vi "Main.vi"() -> ()   [LabVIEW 2017]
doc: "The myRIO Project template acquires acceleration data from the onboard accelerometer and displays the changes of acceleration values in a waveform chart."
uses:
  StateMachineControl.ctl
  <vilib>/Platform/TimedLoop/XDataNode/timing_clust.ctl
  <vilib>/Platform/TimedLoop/XDataNode/nitl_modes.ctl
  <vilib>/Platform/TimedLoop/XDataNode/wakeup.ctl
  <vilib>/robotics/Obstacle Avoidance/Simple Vector Field Histogram/Panic Range.ctl
  <vilib>/myRIO/Instrument Drivers/Onboard IO/DIO/typedefs/DIO Reference.ctl
  <vilib>/myRIO/Common/Instrument Driver Framework/Utilities/typedefs/myRIO Generic Hardware Reference.ctl
  <vilib>/myRIO/Common/Instrument Driver Framework/Utilities/typedefs/Hardware Version Enum.ctl
  <vilib>/myRIO/Common/Instrument Driver Framework/Utilities/typedefs/myRIO v1.0 Reference.ctl
  <vilib>/myRIO/Common/Instrument Driver Framework/Utilities/typedefs/Generic FPGA Reference.ctl
  <vilib>/myRIO/Common/Instrument Driver Framework/myRIO v1.0/DIO/typedefs/DIO Channels List.ctl
  <vilib>/myRIO/Common/Instrument Driver Framework/myRIO v1.0/DIO/typedefs/DIO Channels Enum.ctl
  <vilib>/userdefined/High Color/nirio_resource_hc.ctl
  <vilib>/myRIO/Common/Instrument Driver Framework/myRIO v1.0/Encoder/typedefs/Encoder Signal Mode.ctl
  <vilib>/myRIO/Instrument Drivers/Onboard IO/Encoder/typedefs/Encoder Reference.ctl
  <vilib>/myRIO/Common/Instrument Driver Framework/myRIO v1.0/Encoder/typedefs/Encoder Channels Enum.ctl
  <vilib>/myRIO/Common/Instrument Driver Framework/myRIO v1.0/Encoder/typedefs/Encoder Configuration v1.0.ctl
  <vilib>/myRIO/Instrument Drivers/Onboard IO/PWM/typedefs/PWM Reference.ctl
  <vilib>/myRIO/Common/Instrument Driver Framework/myRIO v1.0/PWM/typedefs/PWM Channels Enum.ctl
  <vilib>/myRIO/Instrument Drivers/Onboard IO/PWM/typedefs/PWM Configuration.ctl
  <vilib>/myRIO/Common/Instrument Driver Framework/Utilities/vis/Is FPGA Ref Available.vi
  <vilib>/myRIO/Common/Instrument Driver Framework/myRIO v1.0/DIO/vis/myRIO v1.1 Open DIO.vi
  <vilib>/myRIO/Instrument Drivers/Onboard IO/DIO/vis/Read.vi
  <vilib>/myRIO/Instrument Drivers/Onboard IO/DIO/vis/Write.vi
  <vilib>/myRIO/Common/Instrument Driver Framework/myRIO v1.0/Encoder/vis/myRIO v1.1 Open Encoder.vi
  <vilib>/myRIO/Instrument Drivers/Onboard IO/Encoder/vis/Read.vi
  <vilib>/myRIO/Common/Instrument Driver Framework/myRIO v1.0/PWM/vis/myRIO v1.1 Open PWM.vi
  <vilib>/myRIO/Instrument Drivers/Onboard IO/PWM/vis/Set Duty Cycle and Frequency.vi
  <vilib>/myRIO/Common/Instrument Driver Framework/Utilities/vis/Validate Channels.vi
  <vilib>/myRIO/Common/Instrument Driver Framework/myRIO v1.0/DIO/vis/myRIO v1.0 Reserve DIO.vi
  <vilib>/myRIO/Common/Instrument Driver Framework/myRIO v1.0/Encoder/vis/myRIO v1.0 Reserve Encoder.vi
  <vilib>/myRIO/Common/Instrument Driver Framework/myRIO v1.0/PWM/vis/myRIO v1.0 Reserve PWM.vi
  <vilib>/myRIO/Common/Instrument Driver Framework/myRIO v1.0/UART/vis/myRIO v1.0 Close UART.vi
  <vilib>/myRIO/Common/Instrument Driver Framework/myRIO v1.0/Resource Manager/vis/myRIO v1.0 Reserve Channel List.vi
  <vilib>/myRIO/Common/Instrument Driver Framework/myRIO v1.0/DIO/vis/myRIO v1.0 Build MUX Configuration DIO.vi
  <vilib>/myRIO/Common/Instrument Driver Framework/myRIO v1.0/Encoder/vis/myRIO v1.0 Build MUX Configuration Encoder.vi
  <vilib>/myRIO/Common/Instrument Driver Framework/myRIO v1.0/PWM/vis/myRIO v1.0 Build MUX Configuration PWM.vi
  <vilib>/myRIO/Common/Instrument Driver Framework/myRIO v1.0/Resource Manager/vis/myRIO v1.0 Reserve Channel.vi
  <vilib>/myRIO/Common/Instrument Driver Framework/myRIO v1.0/Resource Manager/vis/myRIO v1.0 Unreserve Channel.vi
  <vilib>/myRIO/Common/Instrument Driver Framework/myRIO v1.0/Resource Manager/vis/myRIO v1.0 Create Configuration List.vi
  <vilib>/myRIO/Common/Instrument Driver Framework/myRIO v1.0/Resource Manager/vis/myRIO v1.0 Build Mutex Name.vi
  <vilib>/Utility/VariantDataType/GetNumericInfo.vi
  <vilib>/Utility/error.llb/Error Cluster From Error Code.vi
  <vilib>/myRIO/Common/Instrument Driver Framework/myRIO v1.0/myRIO v1.1 Open.vi
  <vilib>/myRIO/Common/Instrument Driver Framework/Utilities/vis/IO Manager.vi
  <vilib>/myRIO/Common/Instrument Driver Framework/Utilities/vis/Configuration Manager.vi
  <vilib>/myRIO/Common/Instrument Driver Framework/myRIO v1.0/Resource Manager/vis/myRIO v1.0 Configure IO.vi
  <vilib>/myRIO/Common/Instrument Driver Framework/myRIO v1.0/myRIO v1.0 Close.vi
  <vilib>/myRIO/Common/Instrument Driver Framework/myRIO v1.0/DIO/vis/myRIO v1.0 Read DIO.vi
  <vilib>/myRIO/Common/Instrument Driver Framework/myRIO v1.0/DIO/vis/myRIO v1.0 Write DIO.vi
  <vilib>/myRIO/Common/Instrument Driver Framework/myRIO v1.0/Encoder/vis/myRIO v1.0 Configure Encoder.vi
  <vilib>/myRIO/Common/Instrument Driver Framework/myRIO v1.0/Encoder/vis/myRIO v1.0 Read Encoder.vi
  <vilib>/myRIO/Common/Instrument Driver Framework/myRIO v1.0/PWM/vis/myRIO v1.0 Write PWM.vi
  <vilib>/myRIO/Common/Instrument Driver Framework/Utilities/vis/FPGA Ref Manager.vi
  <vilib>/myRIO/Common/Instrument Driver Framework/myRIO v1.0/myRIO v1.0 Reset FPGA.vi
  <vilib>/myRIO/Common/Instrument Driver Framework/myRIO v1.0/IRQ/vis/myRIO v1.0 IRQ Info FGV.vi
  <vilib>/myRIO/Common/Instrument Driver Framework/myRIO v1.0/IRQ/vis/myRIO v1.0 Timer IRQ Info FGV.vi
  <vilib>/myRIO/Common/Instrument Driver Framework/myRIO v1.0/IRQ/vis/myRIO v1.0 ISR Agent.vi
  <vilib>/Platform/TimedLoop/XDataNode/XDataNode.xnode
  <vilib>/myRIO/Express VI/Onboard Devices/Button/Button Express VI.xnode
  <vilib>/myRIO/Instrument Drivers/Onboard IO/DIO/vis/myRIO DIO Open.xnode
  <vilib>/myRIO/Express VI/Onboard Devices/LED/LED Express VI.xnode
  <vilib>/myRIO/Express VI/Onboard IO/Encoder/Encoder Express VI.xnode
  <vilib>/myRIO/Common/Instrument Driver Framework/myRIO v1.0/Encoder/typedefs/Encoder Count Direction Enum.ctl
  <vilib>/myRIO/Instrument Drivers/Onboard IO/Encoder/vis/myRIO Encoder Open.xnode
  <vilib>/myRIO/Express VI/Onboard IO/DO/DO Express VI.xnode
  <vilib>/myRIO/Express VI/Onboard IO/PWM/PWM Express VI.xnode
  <vilib>/myRIO/Instrument Drivers/Onboard IO/PWM/vis/myRIO PWM Open.xnode
  <vilib>/myRIO/Instrument Drivers/Utilities/Utilities.lvlib
  <vilib>/myRIO/Instrument Drivers/Onboard IO/Encoder/Encoder.lvlib
  <vilib>/myRIO/Instrument Drivers/Onboard IO/DIO/DIO.lvlib
  <vilib>/myRIO/Instrument Drivers/Onboard IO/PWM/PWM.lvlib
  <vilib>/Platform/TimedLoop/XDataNode/XDNodeRunTimeDep.lvlib
  <vilib>/robotics/Obstacle Avoidance/Simple Vector Field Histogram/NI_Robotics_Simple Vector Field Histogram.lvlib
panel:
  out "obstacle within panic range":bool
  out "histogram":cluster{"Direction":dbl[], dbl[]}[](graph)=[{"Direction"=array[277 elements], [0.5, 0.5, 0.5, 0.5, 0.5, 0.5, 0.5, 0.5, 0.5, 0.5, 0.5, 0.5, 0.5, 0.5, 0.5, 0.5, 0.5, 0.5, 0.5, 0.5, 0.5, 0.5, 0.5, 0.5, 0.5, 0.5, 0.5, 0.5, 0.5, 0.5, 0.5, 0.5, 0.5, 0.5, 0.5, 0.5, 0.5, 0.5, 0.5, 0.5, 0.5, 0.5, 0.5, 0.5, 0.5, 0.5, 0.5, 0.5, 0.5, 0.5, 0.5, 0.5, 0.5, 0.5, 0.5, 0.5, 0.5, 0.5, 0.5, 0.5, 0.5, 0.5, 0.5, 0.5, 0.5, 0.5, 0.5, 0.5, 0.5, 0.5, 0.5, 0.5, 0.5, 0.5, 0.5, 0.5, 0.5, 0.5, 0.5, 0.5, 0.5, 0.5, 0.5, 0.5, 0.5, 0.5, 0.5, 0.5, 0.5, 0.5, 0.5, 0.5, 0.5, 0.5, 0.5, 0.5, 0.5, 0.5, 0.5, 0.5, 0.5, 0.5, 0.5, 0.5, 0.5, 0.5, 0.5, 0.5, 0.5, 0.5, 0.5, 0.5, 0.5, 0.5, 0.5, 0.5, 0.5, 0.5, 0.5, 0.5, 0.5, 0.5, 0.5, 0.5, 0.5, 0.5, 0.5, 0.5, 0.5, 0.5, 0.5, 0.5, 0.5, 0.5, 0.5, 0.5, 0.5, 0.5, 0.5, 0.5, 0.5, 0.5, 0.5, 0.5, 0.5, 0.5, 0.5, 0.5, 0.5, 0.5, 0.5, 0.5, 0.5, 0.5, 0.5, 0.5, 0.5, 0.5, 0.5, 0.5, 0.5, 0.5, 0.5, 0.5, 0.5, 0.5, 0.5, 0.5, 0.5, 0.5, 0.5, 0.5, 0.5, 0.5, 0.5, 0.5, 0.5, 0.5, 0.5, 0.5, 0.5, 0.5, 0.5, 0.5, 0.5, 0.5, 0.5, 0.5, 0.5, 0.5, 0.5, 0.5, 0.5, 0.5, 0.5, 0.5, 0.5, 0.5, 0.5, 0.5, 0.5, 0.5, 0.5, 0.5, 0.5, 0.5, 0.5, 0.5, 0.5, 0.5, 0.5, 0.5, 0.5, 0.5, 0.5, 0.5, 0.5, 0.5, 0.5, 0.5, 0.5, 0.5, 0.5, 0.5, 0.5, 0.5, 0.5, 0.5, 0.5, 0.5, 0.5, 0.5, 0.5, 0.5, 0.5, 0.5, 0.5, 0.5, 0.5, 0.5, 0.5, 0.5, 0.5, 0.5, 0.5, 0.5, 0.5, 0.5, 0.5, 0.5, 0.5, 0.5, 0.5, 0.5, 0.5, 0.5, 0.5, 0.5, 0.5, 0.5, 0.5, 0.5, 0.5, 0.5, 0.5, 0.5, 0.5, 0.5, 0.5, 0.5, 0.5, 0.5, 0.5, 0.5, 0.5, 0.5, 0.5]}, {"Direction"=array[683 elements], [0.0, 1.0, 1.0, 1.0, 1.0, 1.0, 1.0, 1.0, 1.0, 1.0, 1.0, 1.0, 1.0, 1.0, 1.0, 1.0, 1.0, 1.0, 1.0, 1.0, 1.0, 1.0, 1.0, 1.0, 1.0, 1.0, 1.0, 1.0, 1.0, 1.0, 1.0, 1.0, 1.0, 1.0, 1.0, 1.0, 1.0, 1.0, 1.0, 1.0, 1.0, 1.0, 1.0, 1.0, 1.0, 1.0, 1.0, 1.0, 1.0, 1.0, 1.0, 1.0, 1.0, 1.0, 1.0, 1.0, 1.0, 1.0, 1.0, 1.0, 1.0, 1.0, 1.0, 1.0, 1.0, 1.0, 1.0, 1.0, 1.0, 1.0, 1.0, 1.0, 1.0, 1.0, 1.0, 1.0, 1.0, 1.0, 1.0, 1.0, 1.0, 1.0, 1.0, 1.0, 1.0, 1.0, 1.0, 1.0, 1.0, 1.0, 1.0, 1.0, 1.0, 1.0, 1.0, 1.0, 1.0, 1.0, 1.0, 1.0, 1.0, 1.0, 1.0, 1.0, 1.0, 1.0, 1.0, 1.0, 1.0, 1.0, 1.0, 0.0, 0.0, 0.0, 0.0, 0.0, 0.0, 0.0, 0.0, 0.0, 0.0, 0.0, 0.0, 0.0, 0.0, 0.0, 0.0, 0.0, 0.0, 0.0, 0.0, 0.0, 1.0, 1.0, 1.0, 1.0, 1.0, 1.0, 1.0, 1.0, 1.0, 1.0, 1.0, 1.0, 1.0, 1.0, 1.0, 1.0, 1.0, 1.0, 1.0, 1.0, 1.0, 1.0, 1.0, 1.0, 1.0, 1.0, 1.0, 1.0, 1.0, 1.0, 1.0, 1.0, 1.0, 1.0, 1.0, 1.0, 1.0, 1.0, 1.0, 1.0, 1.0, 1.0, 1.0, 1.0, 1.0, 1.0, 1.0, 1.0, 1.0, 1.0, 1.0, 1.0, 1.0, 1.0, 1.0, 1.0, 1.0, 1.0, 1.0, 1.0, 1.0, 1.0, 1.0, 1.0, 1.0, 1.0, 1.0, 1.0, 1.0, 1.0, 1.0, 1.0, 1.0, 1.0, 1.0, 1.0, 1.0, 1.0, 1.0, 1.0, 1.0, 1.0, 1.0, 1.0, 0.0, 0.0, 0.0, 0.0, 0.0, 0.0, 0.0, 0.0, 0.0, 0.0, 0.0, 0.0, 0.0, 0.0, 0.0, 0.0, 0.0, 0.0, 0.0, 0.0, 0.0, 0.0, 0.0, 0.0, 0.0, 0.0, 0.0, 0.0, 0.0, 0.0, 0.0, 0.0, 0.0, 0.0, 0.0, 0.0, 0.0, 0.0, 0.0, 0.0, 0.0, 0.0, 0.0, 0.0, 0.0, 0.0, 0.0, 0.0, 0.0, 0.0, 0.0, 0.0, 0.0, 0.0, 0.0, 0.0, 0.0, 0.0, 0.0, 0.0, 0.0, 0.0, 0.0, 0.0, 0.0, 0.0, 0.0, 0.0, 0.0, 0.0, 0.0, 0.0, 0.0, 0.0, 0.0, 0.0, 0.0, 0.0, 0.0, 0.0, 0.0, 0.0, 0.0, 0.0, 0.0, 0.0, 0.0, 0.0, 0.0, 0.0, 0.0, 0.0, 0.0, 0.0, 0.0, 0.0, 0.0, 0.0, 0.0, 0.0, 0.0, 0.0, 0.0, 0.0, 0.0, 0.0, 0.0, 0.0, 0.0, 0.0, 0.0, 0.0, 0.0, 0.0, 0.0, 0.0, 0.0, 0.0, 0.0, 0.0, 0.0, 0.0, 0.0, 0.0, 0.0, 0.0, 0.0, 0.0, 0.0, 0.0, 0.0, 0.0, 0.0, 0.0, 0.0, 0.0, 0.0, 0.0, 0.0, 0.0, 0.0, 0.0, 0.0, 0.0, 0.0, 0.0, 0.0, 0.0, 0.0, 0.0, 0.0, 0.0, 0.0, 0.0, 0.0, 0.0, 0.0, 0.0, 0.0, 0.0, 0.0, 0.0, 0.0, 0.0, 0.0, 0.0, 0.0, 0.0, 0.0, 0.0, 0.0, 0.0, 0.0, 0.0, 0.0, 0.0, 0.0, 0.0, 0.0, 0.0, 0.0, 0.0, 0.0, 0.0, 0.0, 0.0, 0.0, 0.0, 0.0, 0.0, 0.0, 0.0, 0.0, 0.0, 0.0, 0.0, 0.0, 0.0, 0.0, 0.0, 0.0, 0.0, 0.0, 0.0, 0.0, 0.0, 0.0, 0.0, 0.0, 0.0, 0.0, 0.0, 0.0, 0.0, 0.0, 0.0, 0.0, 0.0, 0.0, 0.0, 0.0, 0.0, 0.0, 0.0, 0.0, 0.0, 0.0, 0.0, 0.0, 0.0, 0.0, 0.0, 0.0, 0.0, 0.0, 0.0, 0.0, 0.0, 0.0, 0.0, 0.0, 0.0, 0.0, 0.0, 0.0, 0.0, 0.0, 0.0, 0.0, 0.0, 0.0, 0.0, 0.0, 0.0, 0.0, 0.0, 0.0, 0.0, 0.0, 0.0, 0.0, 0.0, 0.0, 0.0, 0.0, 0.0, 0.0, 0.0, 0.0, 0.0, 0.0, 0.0, 0.0, 0.0, 0.0, 0.0, 0.0, 1.0, 1.0, 1.0, 1.0, 1.0, 1.0, 1.0, 1.0, 1.0, 1.0, 1.0, 1.0, 1.0, 0.0, 0.0, 0.0, 0.0, 0.0, 0.0, 0.0, 0.0, 0.0, 0.0, 0.0, 0.0, 0.0, 0.0, 0.0, 0.0, 0.0, 0.0, 0.0, 0.0, 0.0, 0.0, 0.0, 0.0, 0.0, 0.0, 0.0, 0.0, 0.0, 0.0, 0.0, 0.0, 0.0, 0.0, 0.0, 0.0, 0.0, 0.0, 0.0, 0.0, 0.0, 0.0, 0.0, 0.0, 0.0, 0.0, 0.0, 0.0, 0.0, 0.0, 0.0, 0.0, 0.0, 0.0, 0.0, 0.0, 0.0, 0.0, 0.0, 0.0, 0.0, 0.0, 0.0, 0.0, 0.0, 1.0, 1.0, 1.0, 1.0, 1.0, 1.0, 1.0, 1.0, 1.0, 1.0, 1.0, 1.0, 1.0, 1.0, 1.0, 1.0, 1.0, 1.0, 1.0, 1.0, 1.0, 1.0, 1.0, 1.0, 1.0, 1.0, 1.0, 1.0, 1.0, 1.0, 1.0, 1.0, 1.0, 1.0, 1.0, 1.0, 1.0, 1.0, 1.0, 1.0, 1.0, 1.0, 1.0, 1.0, 1.0, 1.0, 1.0, 1.0, 1.0, 1.0, 1.0, 1.0, 1.0, 1.0, 1.0, 1.0, 1.0, 1.0, 1.0, 1.0, 1.0, 1.0, 1.0, 1.0, 1.0, 1.0, 1.0, 1.0, 1.0, 1.0, 1.0, 1.0, 1.0, 1.0, 1.0, 1.0, 1.0, 0.0, 0.0, 0.0, 0.0, 0.0, 0.0, 0.0, 0.0, 0.0, 0.0, 0.0, 0.0, 0.0, 0.0, 0.0, 0.0, 0.0, 0.0, 0.0, 0.0, 0.0, 0.0, 0.0, 0.0, 0.0, 0.0, 0.0, 0.0, 0.0, 0.0, 0.0, 0.0, 0.0, 0.0, 0.0]}]
  out "Obs. Avoid. Wall SetPt (m)":dbl
  in  "Min Speed":dbl
  in  "Max Speed":dbl
  out "LIDAR Measured Angle":dbl
  out "intercept":dbl
  out "slope":dbl
  in  "Marked Heading":dbl
  in  "Marked Distance":dbl
  in  "Go!":bool
  in  "Robot Heading":dbl
  out "Pixy Output Array":bool[](array[boolean])
  in  "Length":i32=90
  in  "Starting Index":i32
  out "Indexed Plot":cluster{dbl[], dbl[]}(graph)
  out "XY Graph of LIDAR Data (All Index)":cluster{dbl[], dbl[]}(graph)
  in  "Robot Speed":dbl
  in  "Dist From Wall Setpoint":dbl=0.28
  out "LIDAR LOOP V_RIGHT":dbl
  out "LIDAR LOOP V_LEFT":dbl
  in  "Wall Tracking Boolean":bool
  out "Total Distance Travelled":dbl
  out "LIDAR Right x-avg (m)":dbl
  out "LIDAR Left x-avg (m)":dbl
  out "State":T1
  out "Theta Actual (rad)":dbl
  out "y":dbl
  out "x":dbl
  out "speed setpoint (m/s)":dbl
  out "Output to PWM 2":dbl format="%.2f"
  out "Speed of Motor 2":dbl
  out "Motor 2 Total Distance":dbl
  out "Motor 2 Encoder Count":i32
  out "Counter Direction 2":enum16{"Counting Up", "Counting Down"}(ring)
  out "Overflow? 2":bool
  out "Motor 1 Total Distance":dbl
  out "Output to PWM":dbl format="%.2f"
  out "Speed of Motor 1":dbl
  out "Overflow?":bool
  out "Counter Direction":enum16{"Counting Up", "Counting Down"}(ring)
  out "Motor 1 Encoder Count":i32
  out "Error Out":errorcluster
  in  "Stop":bool
  # "Overview: This LabVIEW project is created to explore and analyse the data output provided by the encoder.\n\nAim of Encoder Data Analysis\n1. Process the number of counts generated by the encoder as the input.\n2. Output the motor speed and distance travelled."
  # "Motor 1"
  # "Motor 1 Encoder"
  # "Note: distance is in (m)"
  # "Note: speed is in (m/s)"
  # "Motor 2"
  # "Motor 2 Encoder"
  # "Note: speed is in (m/s)"
  # "Robot Control"
  # "Distance in m."
  # "Heading in (deg)."
  # "Speed is in m/s."
  # "Robot Position"
  # "Measured Using Index 0-90"
  # "Colour Sensor"
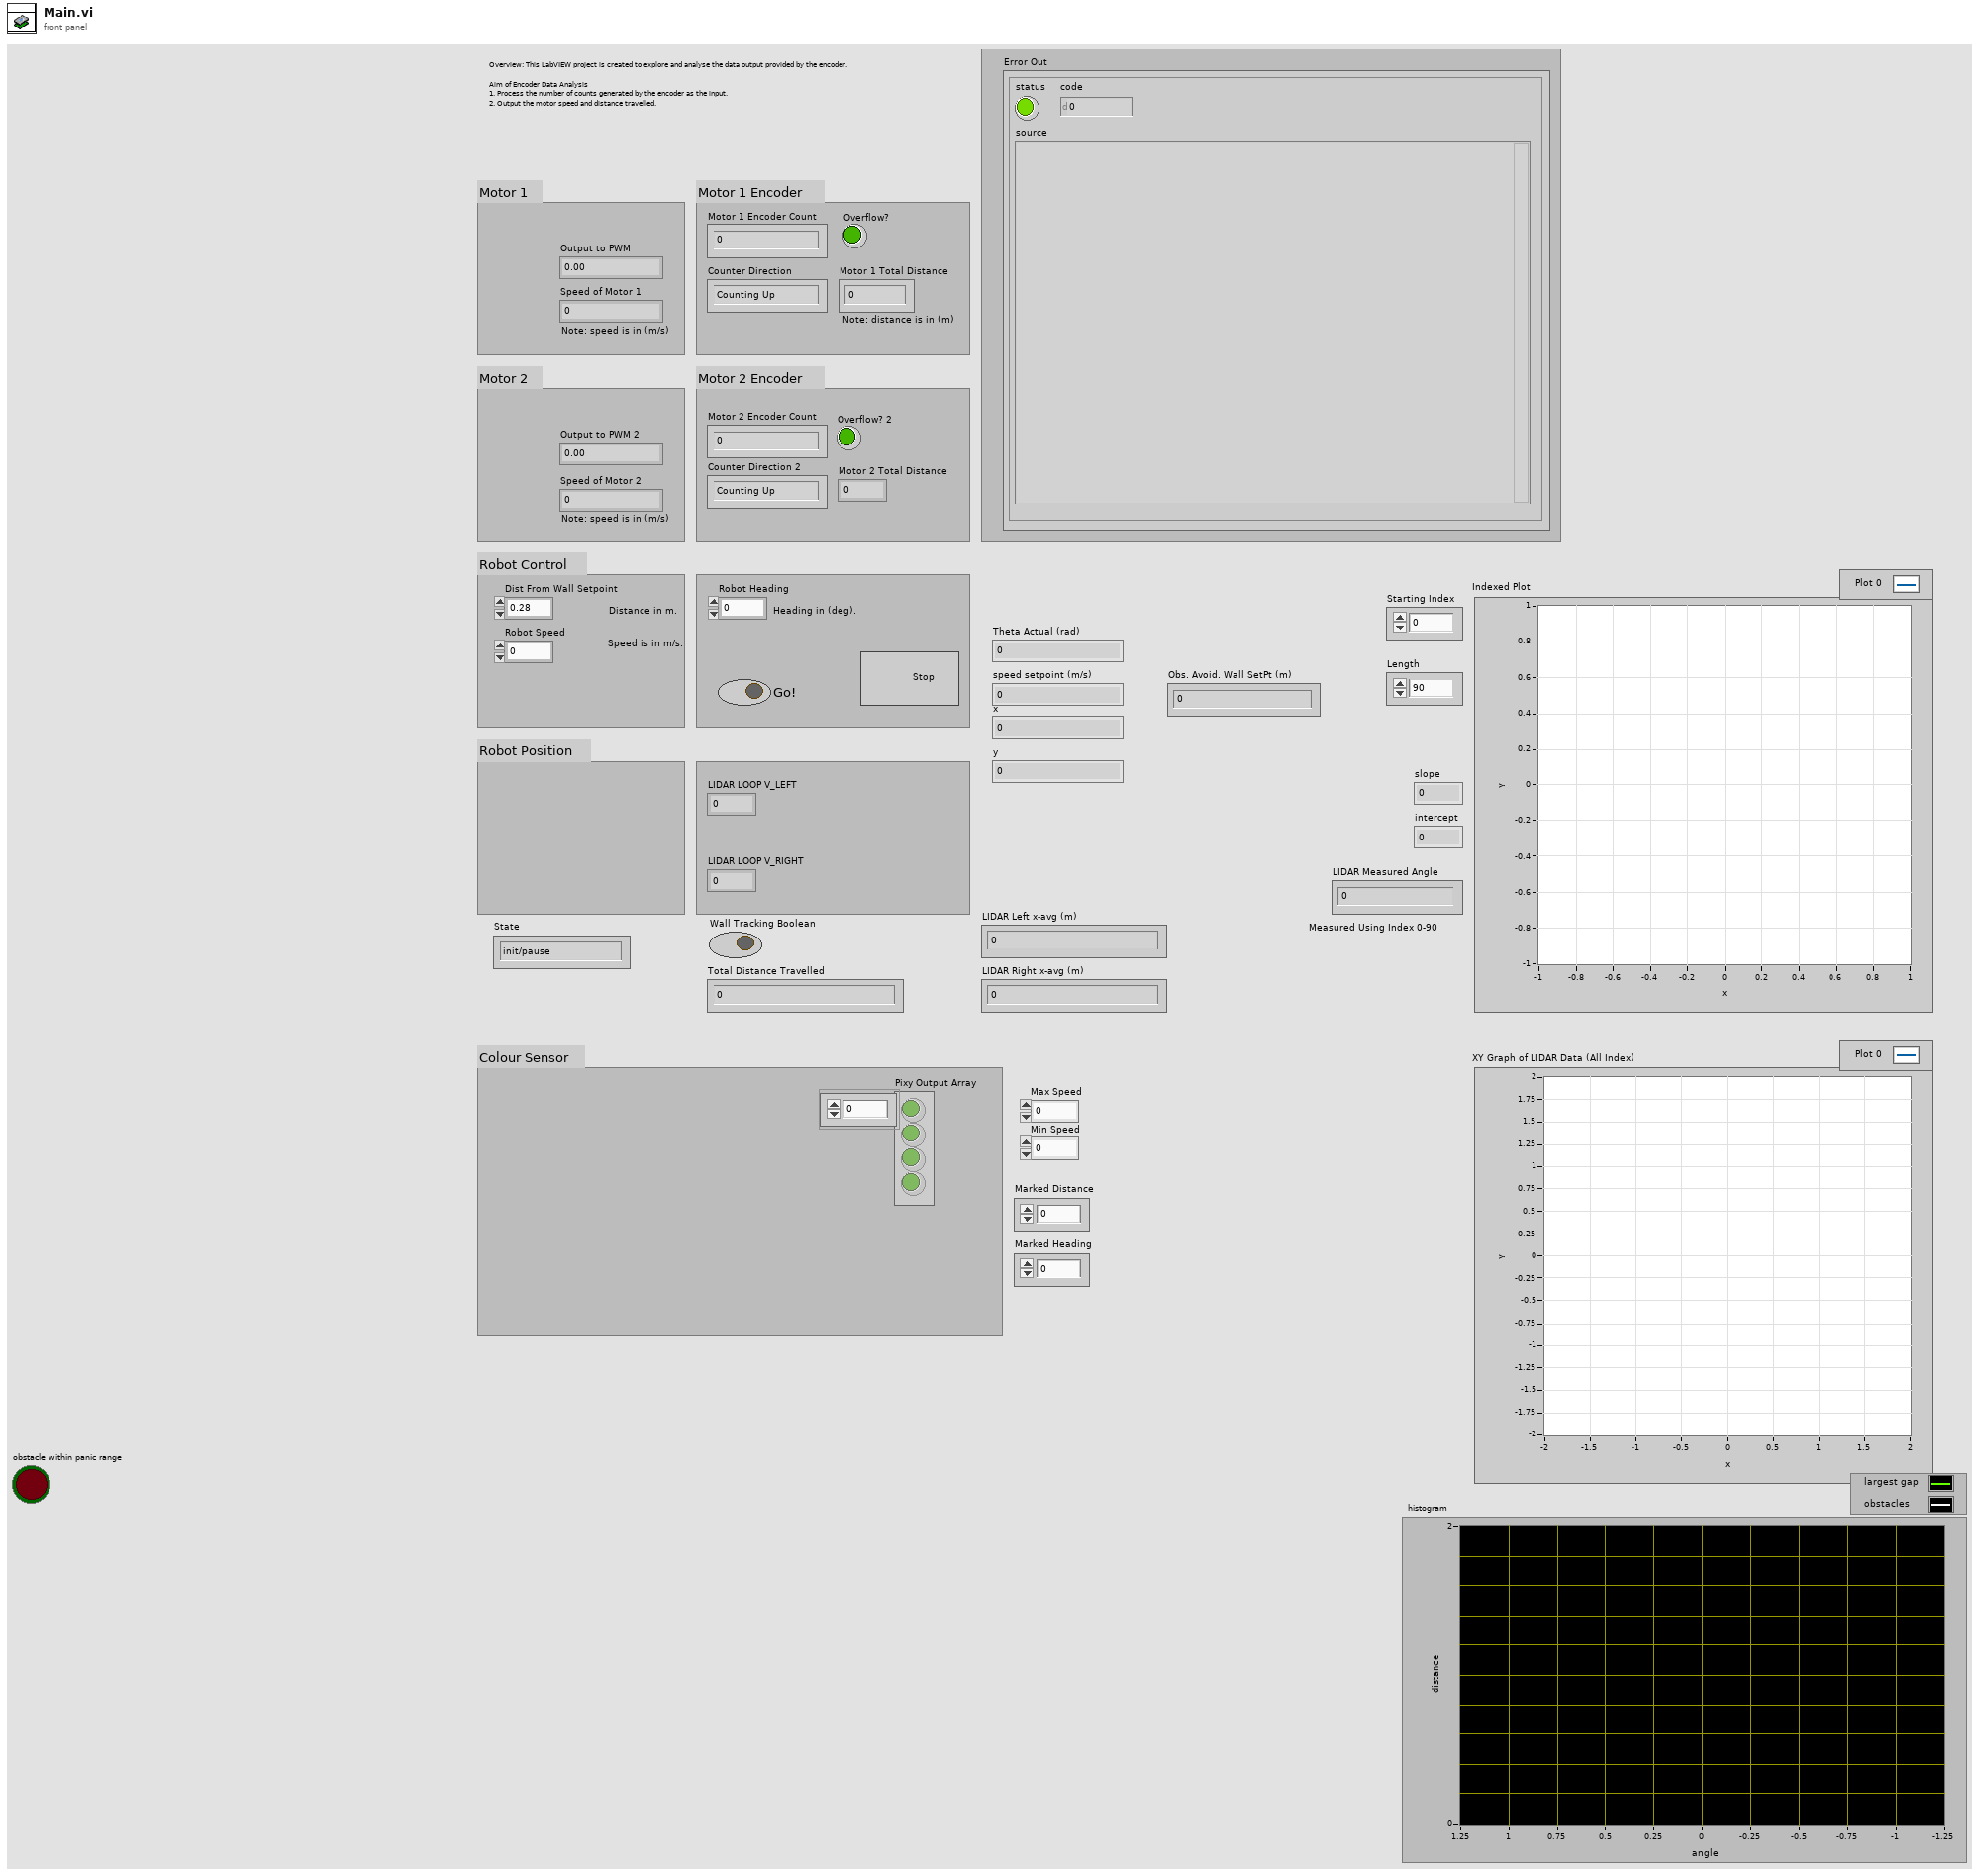
[diagram p1: front panel]
types:
  T1 = typedef "StateMachineControl.ctl" = enum16{"init/pause", "wall tracking w/ obs avoidance", "yellow zig-zag", "blue uneven surface", "red ramp", "green prepare to stop", "note down current distance", "go forward fixed dist & continue", "go forward fixed dist & stop", "stop finite state machine", "stop robot"}
  T2 = typedef "XDNodeRunTimeDep.lvlib/timing_clust.ctl" = cluster{"Expected End [f-1]":u64, "Actual End [f-1]":u64, "Finished Late? [f-1]":bool, "Expected End [i-1]":u64, "Actual End [i-1]":u64, "Finished Late? [i-1]":bool, "Expected Start [i]":u64, "Actual Start [i]":u64, "Expected Start [f]":u64, "Actual Start [f]":u64, "Source Name":string, "Structure Name":string, "Period":i64, "Deadline":i64, "Offset":i64, "Start":i64, "Priority":i32, "Timeout":i32, "Mode":T3, "Wakeup Reason":T4, "Error":errorcluster, "Source Type":string, "Secondary Source Type":string, "Global End Time":u64, "Global Start Time":u64, "Frame Duration":u64, "Iteration Duration":u64, "Assigned CPU":i32, "I/O Scan Engine Mode":u32}
  T3 = typedef "XDNodeRunTimeDep.lvlib/nitl_modes.ctl" = enum32{"No Change", "Process missed periods, maintain original phase", "Discard missed periods, maintain original phase", "Process missed periods, ignore original phase", "Discard missed periods, ignore original phase"}
  T4 = typedef "XDNodeRunTimeDep.lvlib/wakeup.ctl" = enum32{"Normal", "Aborted", "Asynchronous wakeup", "Timing source error", "Timed loop error", "Timeout"}
  T5 = typedef "DIO.lvlib/DIO Reference.ctl" = cluster{"myRIO Reference":T6, "DIO Channels List":T10}
  T6 = typedef "myRIO Generic Hardware Reference.ctl" = cluster{"myRIO Model":T7, "myRIO Hardware Reference":T8}
  T7 = typedef "Hardware Version Enum.ctl" = enum16{"Unknown", "myRIO-1900", "myRIO-1950", "roboRIO", "NI ELVIS RIO CM"}
  T8 = typedef "myRIO v1.0 Reference.ctl" = cluster{"Generic FPGA Reference":T9, "Allow multiple opens":bool}
  T9 = typedef "Generic FPGA Reference.ctl" = refnum<k20>
  T10 = typedef "DIO Channels List.ctl" = T11[]
  T11 = typedef "DIO Channels Enum.ctl" = enum16{"Not Connected", "C/DIO0", "C/DIO1", "C/DIO2", "C/DIO3", "C/DIO4", "C/DIO5", "C/DIO6", "C/DIO7", "A/DIO0", "A/DIO1", "A/DIO2", "A/DIO3", "A/DIO4", "A/DIO5", "A/DIO6", "A/DIO7", "A/DIO8", "A/DIO9", "A/DIO10", "A/DIO11", "A/DIO12", "A/DIO13", "A/DIO14", "A/DIO15", "B/DIO0", "B/DIO1", "B/DIO2", "B/DIO3", "B/DIO4", "B/DIO5", "B/DIO6", "B/DIO7", "B/DIO8", "B/DIO9", "B/DIO10", "B/DIO11", "B/DIO12", "B/DIO13", "B/DIO14", "B/DIO15", "LED0", "LED1", "LED2", "LED3", "Button0", "DIO/DIO0", "DIO/DIO1", "DIO/DIO2", "DIO/DIO3", "DIO/DIO4", "DIO/DIO5", "DIO/DIO6", "DIO/DIO7", "DIO/DIO8", "DIO/DIO9", "SPI/CS0", "SPI/CS1", "SPI/CS2", "SPI/CS3", "LED RADIO (Green)", "LED RADIO (Red)", "LED COMM (Green)", "LED COMM (Red)", "LED MODE (Green)", "LED MODE (Red)"}
  T12 = typedef "nirio_resource_hc.ctl" = tag
  T13 = typedef "NI_Robotics_Simple Vector Field Histogram.lvlib/Panic Range.ctl" = cluster{"panic threshold distance (0)":dbl, "panic threshold angle (0)":dbl}
  T14 = typedef "PWM.lvlib/PWM Reference.ctl" = cluster{"myRIO Reference":T6, "PWM Channels Enum":T15, "PWM Configuration":T16}
  T15 = typedef "PWM Channels Enum.ctl" = enum16{"Not Connected", "C/PWM0", "C/PWM1", "A/PWM0", "A/PWM1", "A/PWM2", "B/PWM0", "B/PWM1", "B/PWM2", "PWM/PWM0", "PWM/PWM1", "PWM/PWM2", "PWM/PWM3", "PWM/PWM4", "PWM/PWM5", "PWM/PWM6", "PWM/PWM7", "PWM/PWM8", "PWM/PWM9"}
  T16 = typedef "PWM.lvlib/PWM Configuration.ctl" = cluster{"Frequency":dbl, "Duty Cycle":dbl}
  T17 = typedef "Encoder.lvlib/Encoder Reference.ctl" = cluster{"myRIO Reference":T6, "Encoder Channels Enum":T18}
  T18 = typedef "Encoder Channels Enum.ctl" = enum16{"Not Connected", "C/ENC0", "C/ENC1", "A/ENC", "B/ENC", "DIO/ENC0", "DIO/ENC1", "DIO/ENC2", "DIO/ENC3", "DIO/ENC4"}
  T19 = typedef "Encoder Signal Mode.ctl" = enum16{"Quadrature phase signal", "Step and direction signal"}
  T20 = typedef "NI_Robotics_Simple Vector Field Histogram.lvlib/Gap Description.ctl" = cluster{"angle to gap":dbl, "size of gap":dbl}
  T21 = typedef "Encoder Count Direction Enum.ctl" = enum16{"Counting Up", "Counting Down"}
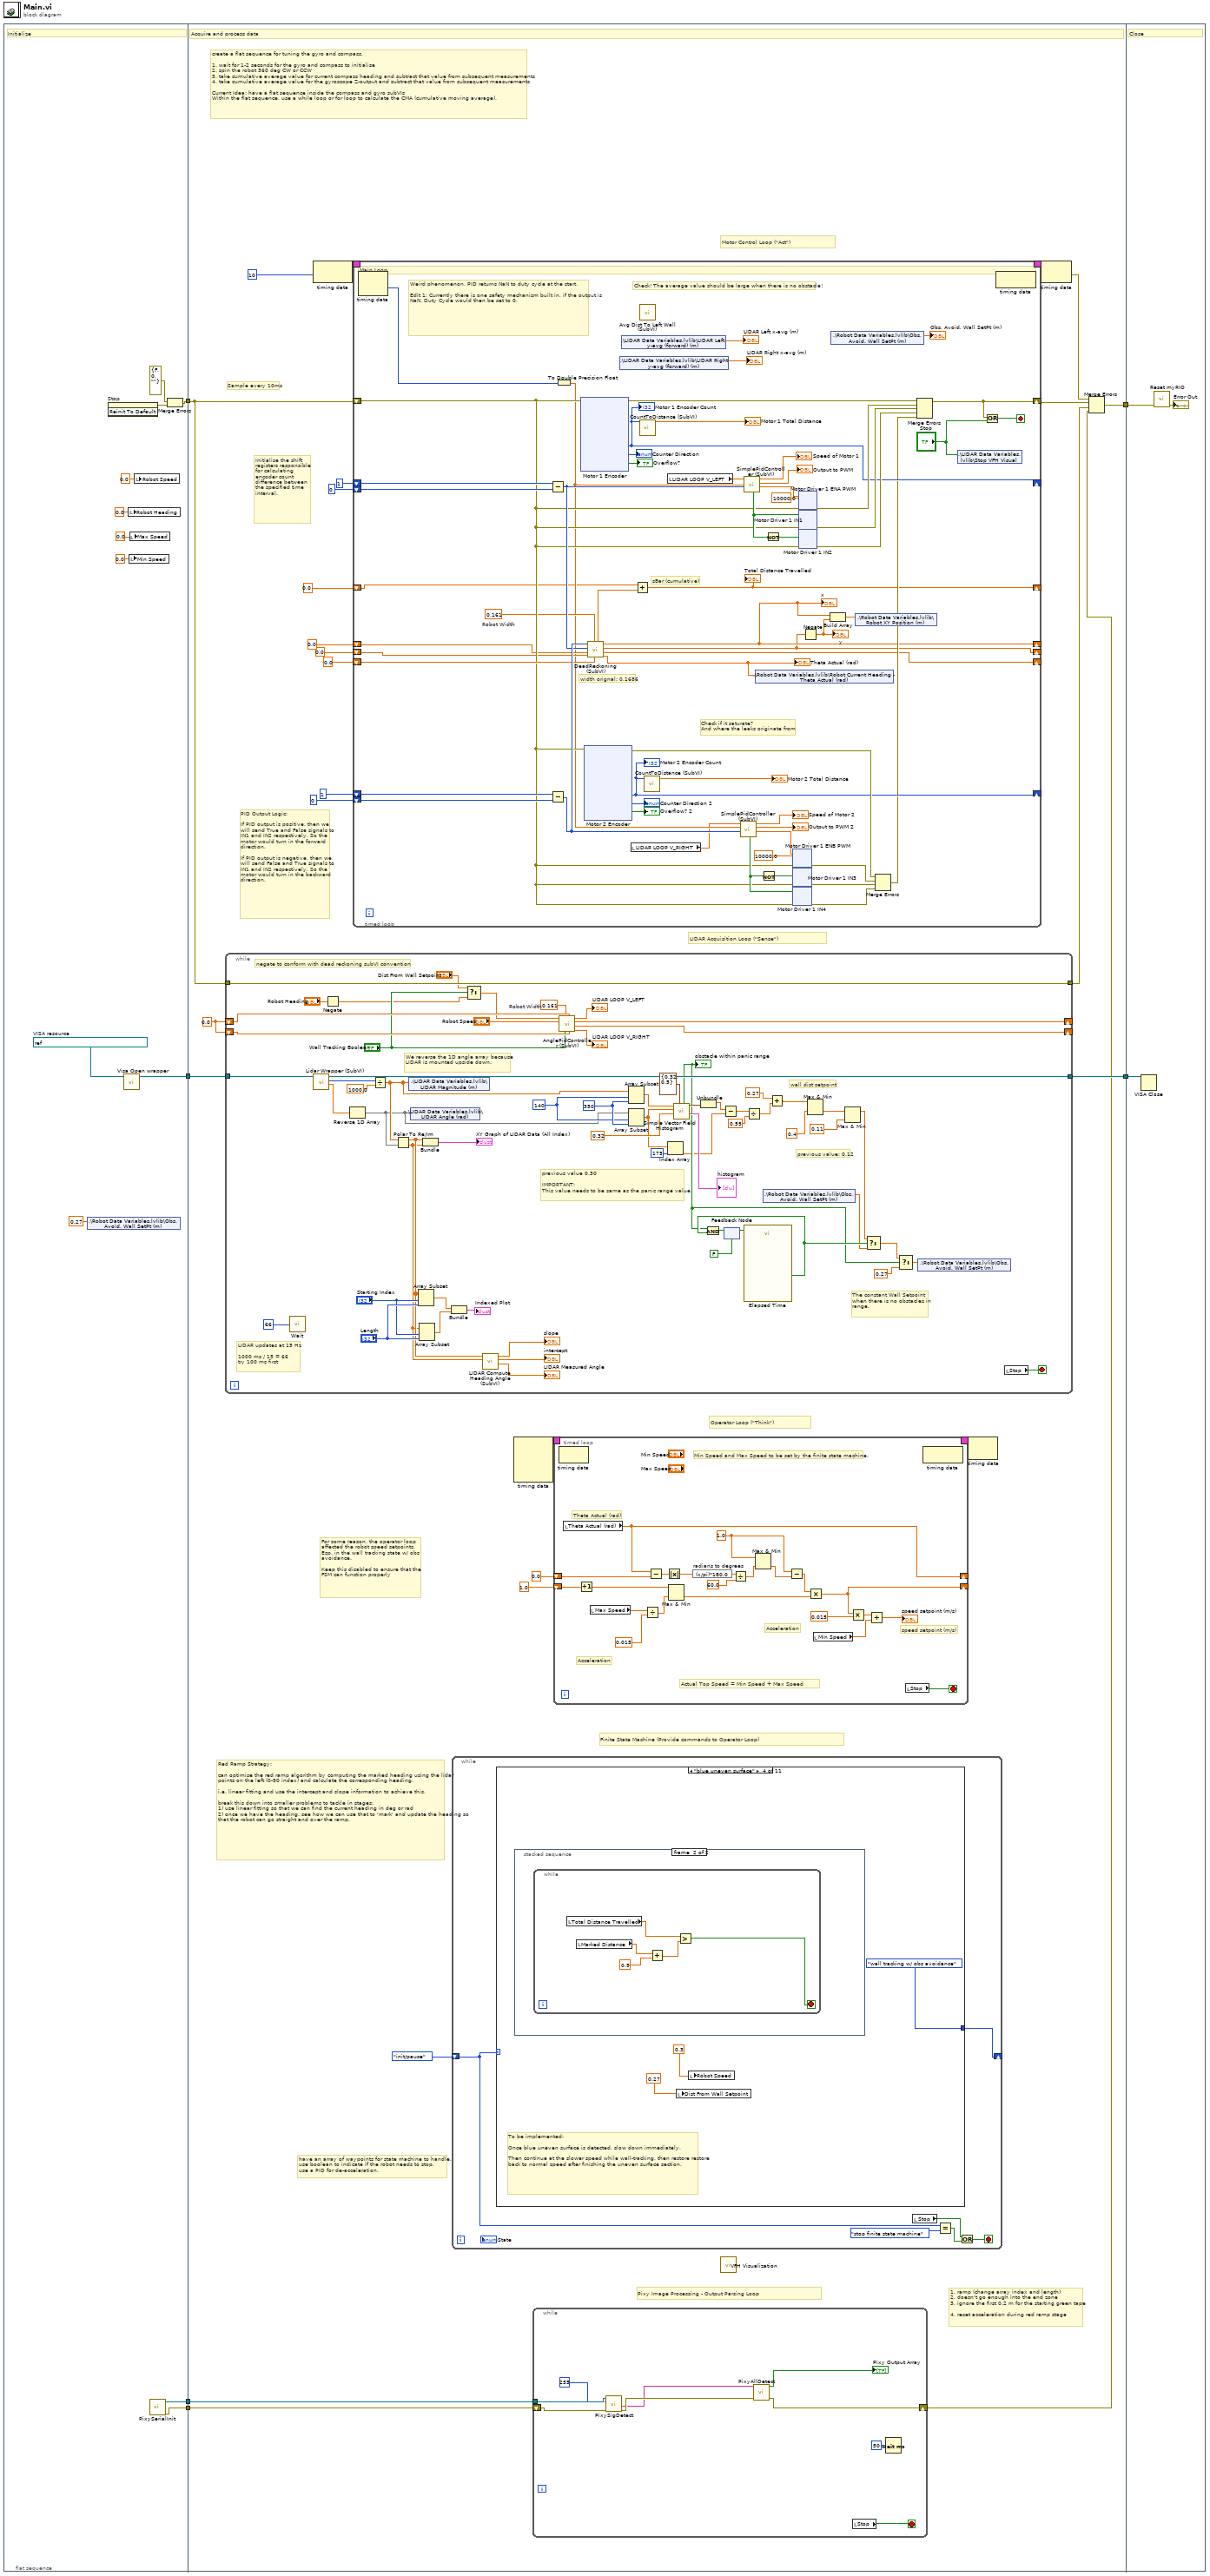
[diagram p0: block diagram]
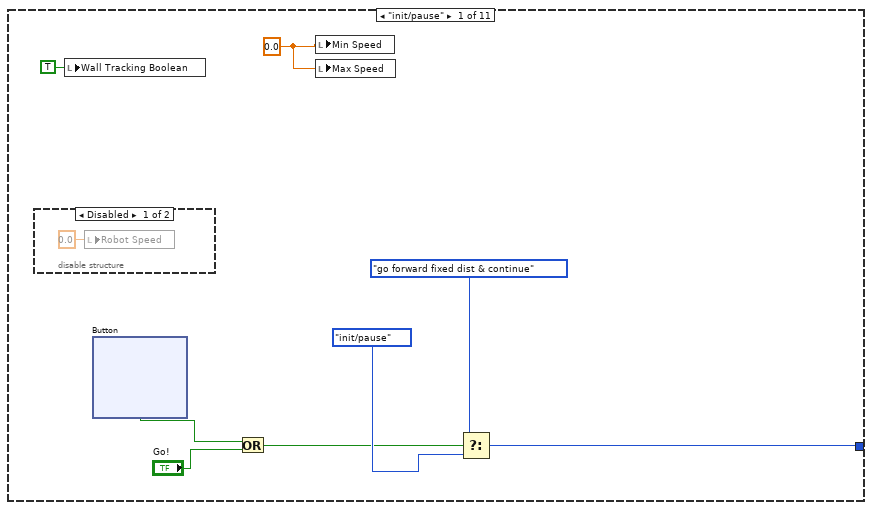
[diagram p2: hidden frame]
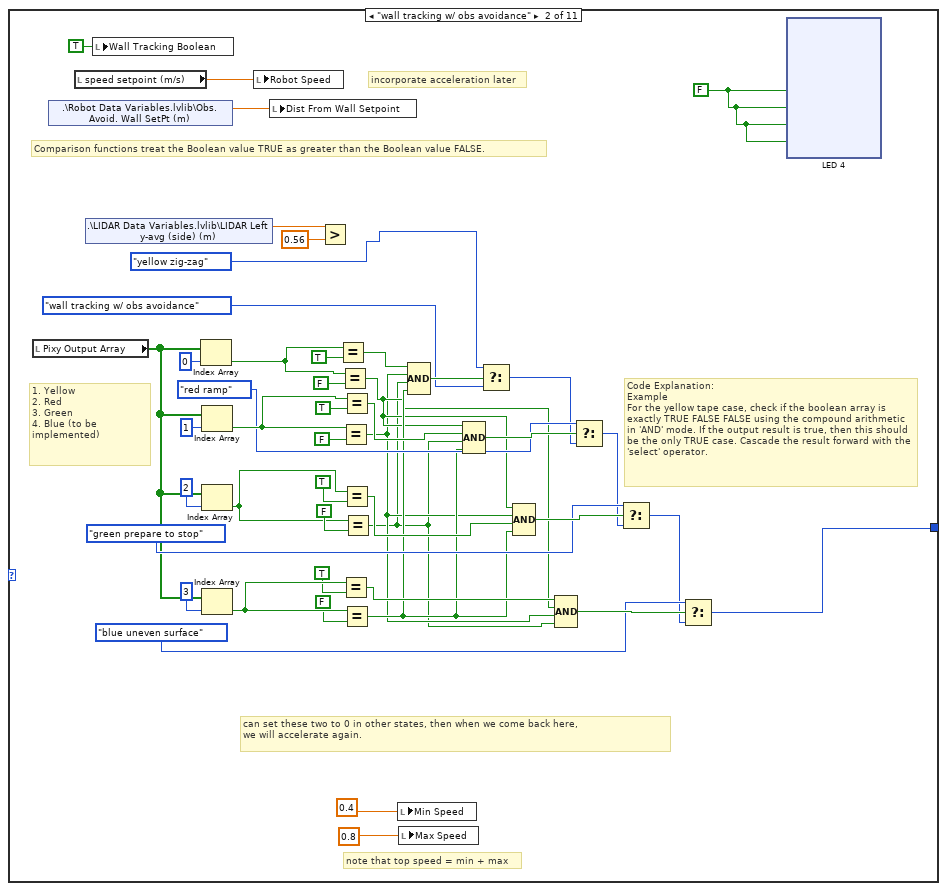
[diagram p4: hidden frame]
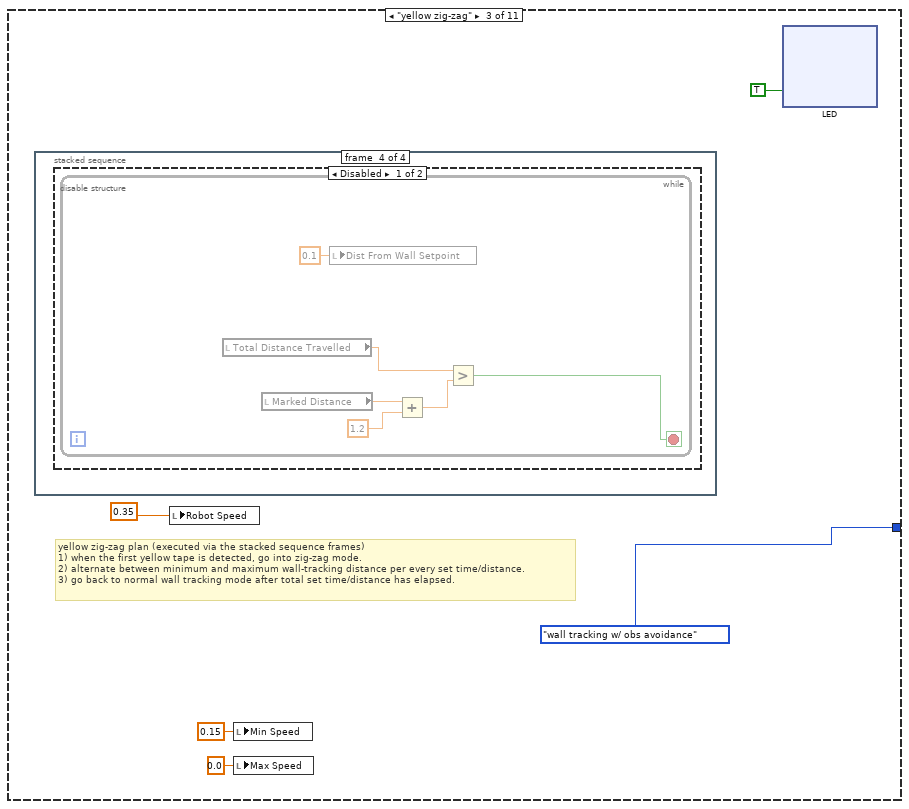
[diagram p5: hidden frame]
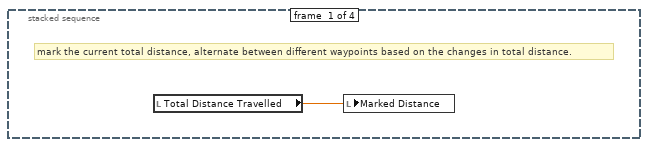
[diagram p6: hidden frame]
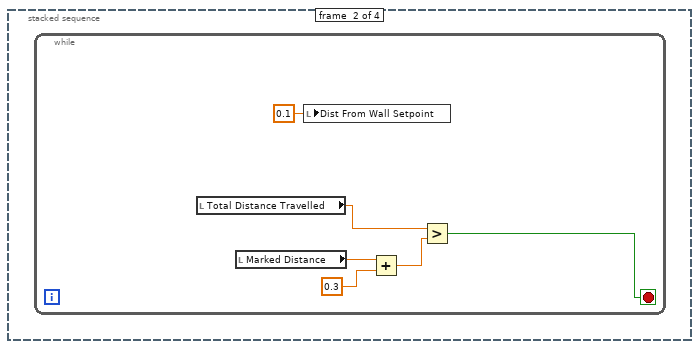
[diagram p7: hidden frame]
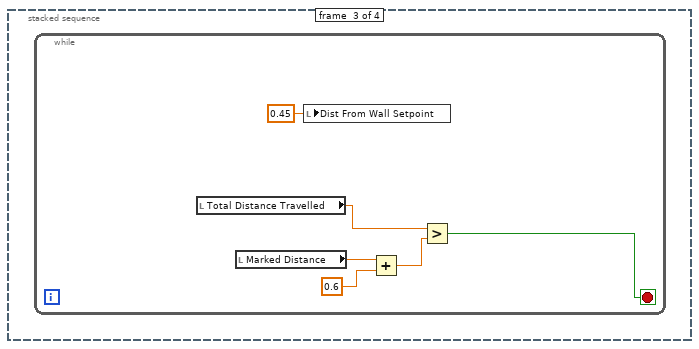
[diagram p8: hidden frame]
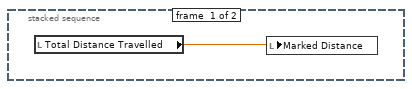
[diagram p10: hidden frame]
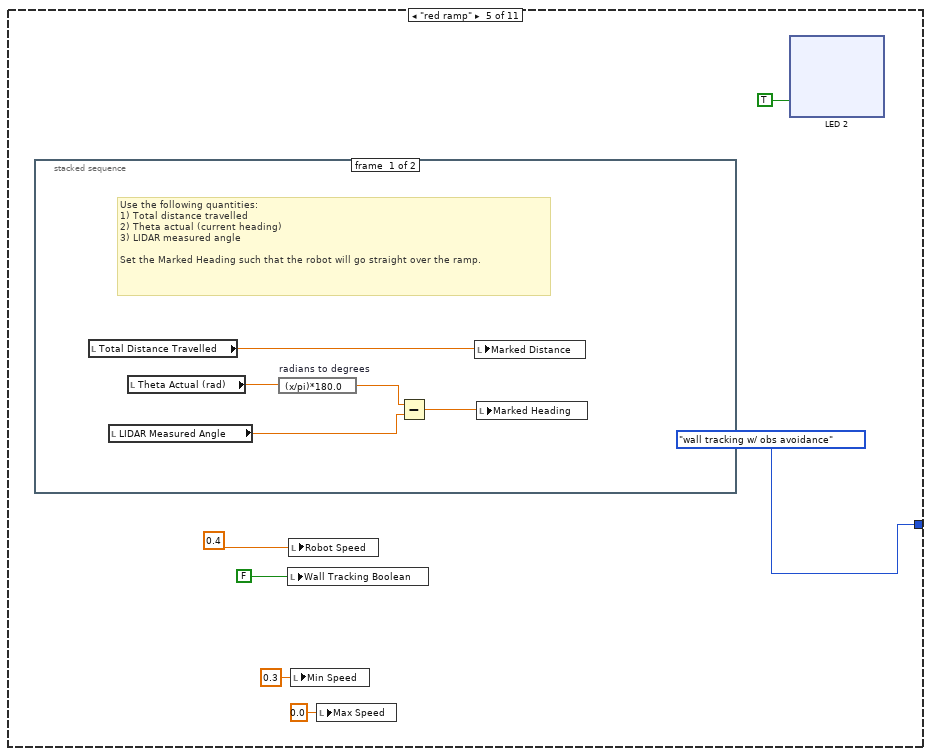
[diagram p11: hidden frame]
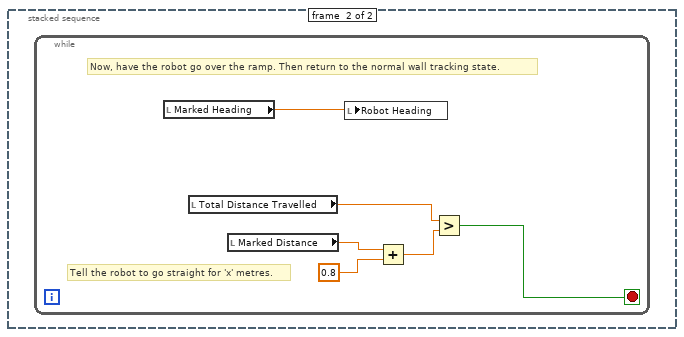
[diagram p12: hidden frame]
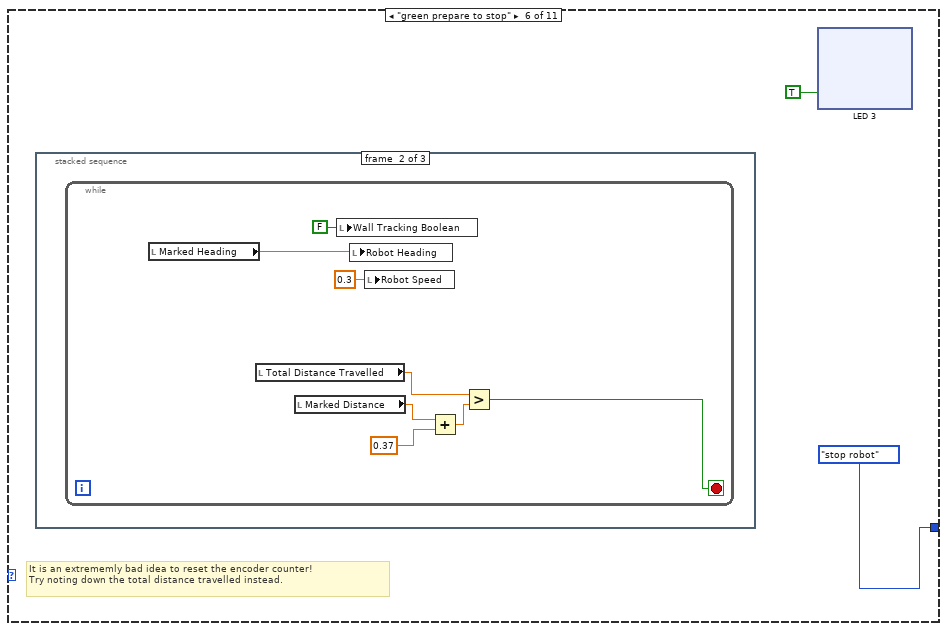
[diagram p13: hidden frame]
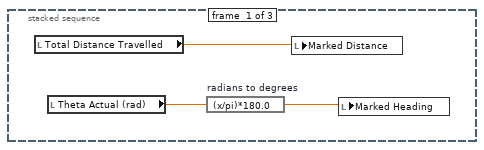
[diagram p14: hidden frame]
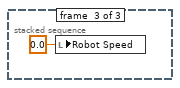
[diagram p15: hidden frame]
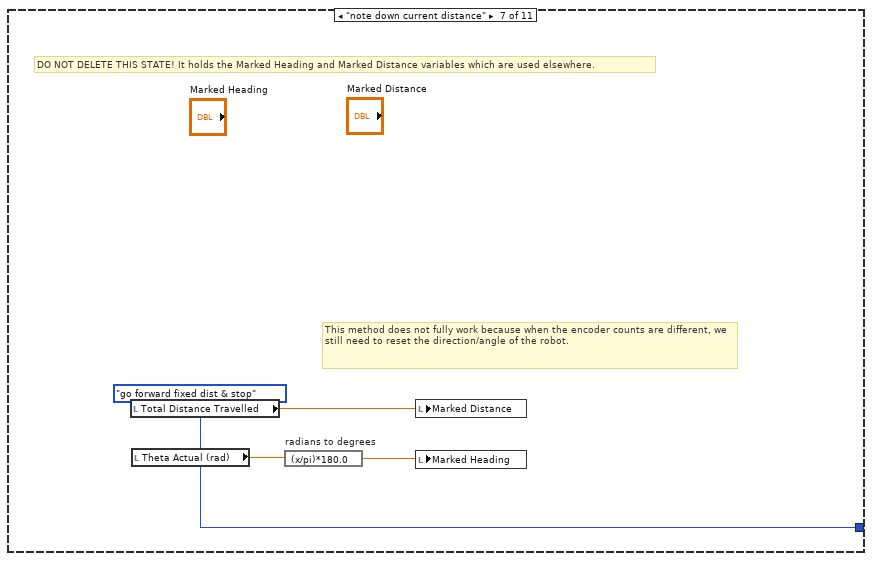
[diagram p16: hidden frame]
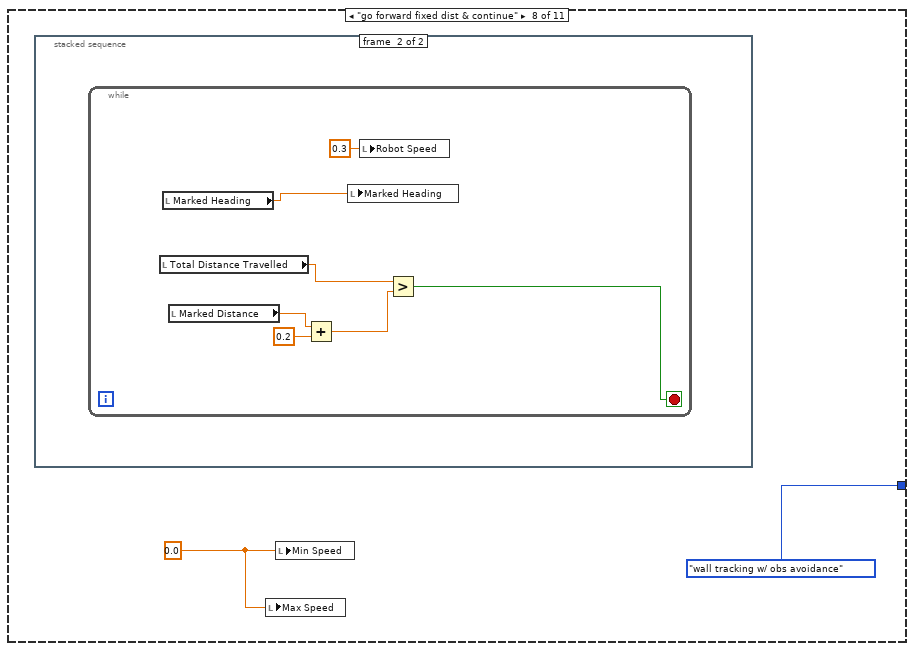
[diagram p17: hidden frame]
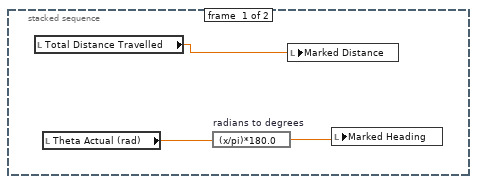
[diagram p18: hidden frame]
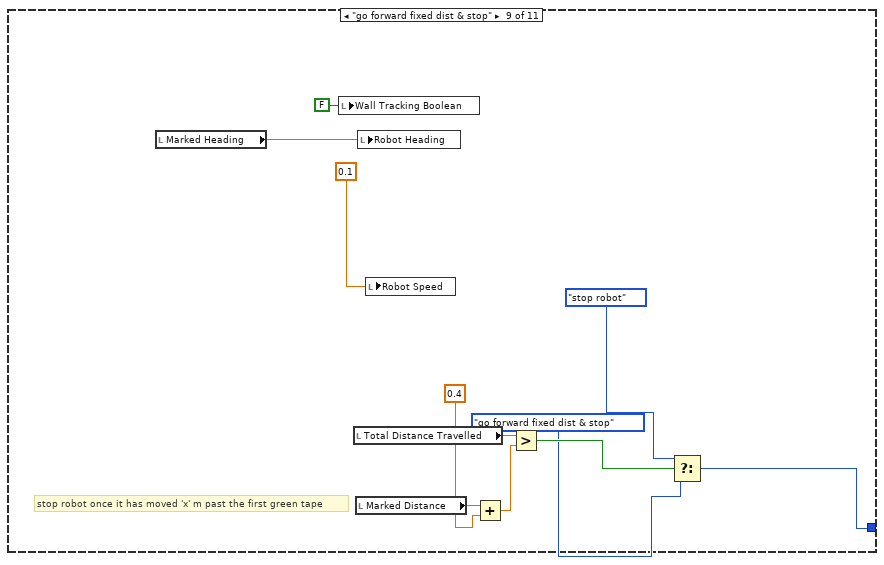
[diagram p19: hidden frame]
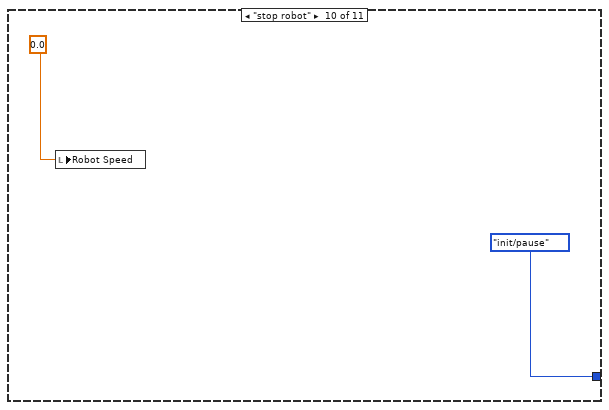
[diagram p20: hidden frame]
diagram:
  n1 = flat-sequence {
    tunnel: [w17] -> w6
    tunnel: [w15] -> w4
    tunnel: [w13] -> w2
    tunnel: [w12] -> w1
    tunnel: w6 -> [w31]
    tunnel: [w42] -> w5
    tunnel: w4 -> [w33]
    tunnel: [w32] -> w3
    tunnel: w2 -> [w26]
    tunnel: w1 -> [w25]
    tunnel: w5 -> [w846]
    tunnel: w3 -> [w847]
    frame #0 {
      w16 = refnum<visa-resource-name> "TCPIP::169.254.233.170::2112::SOCKET"  # VISA resource
      # "Initialize"
      n2 = shared-variable ".\\Robot Data Variables.lvlib\\Obs. Avoid. Wall SetPt (m)"(0.27 ("Obs. Avoid. Wall SetPt (m)")) -> ()  [unwired: 1 in, 1 out]
      n3 = invoke on="Stop" class="Bool (strict)" method="Reinit To Default"() -> (error out=w14:errorcluster)  [unwired: 3 in, 2 out]
      n4 = call "Visa Open wrapper.vi"("VISA resource"=w16) -> ("VISA resource name out"=w15:refnum<visa-resource-name>)  [unwired: 10 in]
      n5 = local write "Robot Heading"(0.0 ("Robot Heading")) -> ()
      n6 = local write "Min Speed"(0.0 ("Min Speed")) -> ()
      n7 = local write "Max Speed"(0.0 ("Max Speed")) -> ()
      n8 = local write "Robot Speed"(0.0 ("Robot Speed")) -> ()
      n9 = call "PixySerialInit.vi"() -> ("error out"=w12:errorcluster, "VISA resource name out"=w13:refnum<visa-resource-name>)  [unwired: 10 in]
      n10 = Merge Errors(errorcluster {"status"=FALSE, "code"=0, "source"=""} ("error in (no error)"), w14) -> (w17:errorcluster)
    }
    frame #1 {
      w19 = 0.0 ("Current Error")
      # "1. ramp (change array index and length)\n2. doesn't go enough into the end zone\n3. ignore the first 0.2 m for the starting green tape\n\n4. reset acceleration during red ramp stage"
      # "Operator Loop (\"Think\")"
      # "Red Ramp Strategy:\n\ncan optimise the red ramp algorithm by computing the marked heading using the lidar points on the left (0-90 index) and calculate the corresponding heading.\n\ni.e. linear fitting and use the intercept and slope information to achieve this. \n\nbreak this down into smaller problems to tackle in stages:\n1) use linear fitting so that we can find the current heading in deg or rad\n2) once we have the heading, see how we can use that to 'mark' and update the heading so that the robot can go straight and over the ramp."
      # "For some reason, the operator loop affected the robot speed setpoints.\nEsp. in the wall tracking state w/ obs avoidance.\n\nKeep this disabled to ensure that the FSM can function properly"
      # "Pixy Image Processing - Output Parsing Loop"
      # "Finite State Machine (Provide commands to Operator Loop)"
      # "create a flat sequence for tuning the gyro and compass.\n\n1. wait for 1-2 seconds for the gyro and compass to initialise\n2. spin the robot 360 deg CW or CCW\n3. take cumulative average value for current compass heading and subtract that value from subsequent measurements\n4. take cumulative average value for the gyroscope Z-output and subtract that value from subsequent measurements\n\nCurrent Idea: have a flat sequence inside the compass and gyro subVIs\nWithin the flat sequence, use a while loop or for loop to calculate the CMA (cumulative moving average)."
      # "have an array of waypoints for state machine to handle,\nuse boolean to indicate if the robot needs to stop,\nuse a PID for de-acceleration."
      # "LIDAR Acquisition Loop (\"Sense\")"
      # "Motor Control Loop (\"Act\")"
      # "PID Output Logic:\n\nIf PID output is positive, then we will send True and False signals to IN1 and IN2 respectively. So the motor would turn in the forward direction.\n\nIf PID output is negative, then we will send False and True signals to IN1 and IN2 respectively. So the motor would turn in the backward direction."
      # "Initialise the shift registers responsible for calculating encoder count difference between the specified time interval."
      # "Sample every 10ms"
      # "Acquire and process data"
      n11 = while {
        tunnel: w33 -> [w476]
        tunnel: [w475] -> w32
        tunnel: w31 -> [w471]
        tunnel: [w471] -> w30
        shift-right: [w470] -> _
        shift-left: w19 -> [w468]
        shift-right: [w469] -> _
        shift-left: w19 -> [w467]
        stop <- w472 stop-if-true
        w437 = 140 ("length")
        w440 = 350 ("length")
        w464 = 0.161  # Robot Width
        # "wall dist setpoint"
        # "The constant Wall Setpoint when there is no obstacles in range."
        # "previous value 0.30\n\nIMPORTANT:\nThis value needs to be same as the panic range value."
        # "previous value: 0.12"
        # "negate to conform with dead reckoning subVI convention"
        # "We reverse the 1D angle array because LIDAR is mounted upside down."
        # "LIDAR updates at 15 Hz\n\n1000 ms / 15 = 66\ntry 100 ms first"
        n12 = call "Wait"("Count(mSec)"=u32 66) -> ()  [unwired: 1 out]
        n13 = call "Lidar Wrapper (SubVI).vi"("VISA Refnum in"=w476) -> ("Array"=w460:dbl[], "Distance Array"=w459:u32[], "VISA Refnum out"=w475:refnum<visa-resource-name>)  [unwired: 8 in]
        n14 = Negate(x="Robot Heading") -> (-x=w452:dbl)
        n15 = Reverse 1D Array(array=w460) -> (reversed array=w421:dbl[])
        n16 = Divide(x=w459, y=1000.0) -> (x/y=w423:dbl[])
        n17 = Polar To Re/Im(2:w421, 3:w423) -> (0:w447:dbl[], 1:w448:dbl[])
        n18 = shared-variable ".\\LIDAR Data Variables.lvlib\\LIDAR Magnitude (m)"(w423) -> ()  [unwired: 1 in, 1 out]
        n19 = shared-variable ".\\LIDAR Data Variables.lvlib\\LIDAR Angle (rad)"(w421) -> ()  [unwired: 1 in, 1 out]
        n20 = Array Subset(array=w448, index="Starting Index", length="Length") -> (w451:dbl[])
        n21 = Array Subset(array=w447, index="Starting Index", length="Length") -> (w450:dbl[])
        n22 = Bundle(w448, w447) -> (→"XY Graph of LIDAR Data (All Index)":cluster{dbl[], dbl[]})  [unwired: 1 in]
        n23 = Bundle(w451, w450) -> (→"Indexed Plot":cluster{dbl[], dbl[]})  [unwired: 1 in]
        n24 = Select(t="Dist From Wall Setpoint", s="Wall Tracking Boolean", f=w452) -> (s? t:f=w453:dbl)
        n25 = call "LIDAR Compute Heading Angle (SubVI).vi"("Y Array"=w447, "X Array"=w448) -> ("LIDAR Computed Angle"=→"LIDAR Measured Angle":dbl, "intercept"=→"intercept":dbl, "slope"=→"slope":dbl)  [unwired: 7 in]
        n26 = call "AnglePidController (SubVI).vi"("Sum Error"=w467, "Previous Error"=w468, "Wall Tracking Boolean"="Wall Tracking Boolean", "Robot Width (m)"=w464, "Desired Speed (m|s)"="Robot Speed", "PID Setpoint [Wall Distance (m) OR Heading (deg)]"=w453) -> ("Velocity Right (m|s)"=→"LIDAR LOOP V_RIGHT":dbl, "Sum For Shift Register"=w469:dbl, "Current Error"=w470:dbl, "Velocity Left (m|s)"=→"LIDAR LOOP V_LEFT":dbl)  [unwired: 2 in]
        n27 = Array Subset(array=w423, index=w437, length=w440) -> (w422:dbl[])
        n28 = Array Subset(array=w421, index=w437, length=w440) -> (w414:dbl[])
        n29 = Index Array(array=w414, index=175) -> (element=w420:dbl)
        n30 = call <vilib>:"Simple Vector Field Histogram.vi"("panic range"=T13 {"panic threshold distance (0)"=0.32, "panic threshold angle (0)"=0.5}, "distance threshold"=0.32, "direction angles"=w414, "distances"=w422) -> ("histogram"=→"histogram":cluster{"Direction":dbl[], dbl[]}[], "largest gap"=w444:T20, "obstacle within panic range"=w424:bool)  [unwired: 3 in, 2 out]
        "obstacle within panic range" <- w424
        n31 = Unbundle(w444) -> ("angle to gap"=w438:dbl)  [unwired: 1 out]
        n32 = Subtract(x=w438, y=w420) -> (x-y=w436:dbl)
        n33 = feedback #1(FALSE) -> (w431:bool)
        n34 = call "Elapsed Time"("Reset"=w431) -> ("Time has Elapsed"=w430:bool)  [unwired: 11 in, 7 out]
        n35 = And(x=w424, y=w430) -> (x .and. y?=w432:bool)
        n36 = feedback-in #1(w432) -> ()
        n37 = Divide(x=w436, y=0.55) -> (x/y=w435:dbl)
        n38 = shared-variable ".\\Robot Data Variables.lvlib\\Obs. Avoid. Wall SetPt (m)"() -> (w429:dbl)  [unwired: 1 in, 1 out]
        n39 = Add(x=0.27 ("t"), y=w435) -> (x+y=w416:dbl)
        n40 = Max & Min(x=w416, y=0.4) -> (min(x,y)=w418:dbl)  [unwired: 1 out]
        n41 = Max & Min(x=w418, y=0.11 ("t")) -> (max(x,y)=w415:dbl)  [unwired: 1 out]
        n42 = Select(t=w415, s=w430, f=w429) -> (s? t:f=w427:dbl)
        n43 = Select(t=w427, s=w424, f=0.27 ("Obs. Avoid. Wall SetPt (m)")) -> (s? t:f=w425:dbl)
        n44 = shared-variable ".\\Robot Data Variables.lvlib\\Obs. Avoid. Wall SetPt (m)"(w425) -> ()  [unwired: 1 in, 1 out]
        n45 = local read "Stop"() -> (w472:bool)
      }
      n46 = node-c288(i64 10 ("Period")) -> (w45:T2)
      n47 = timed-loop {
        shift-right: [w531] -> w40
        shift-left: w31 -> [w498]
        timing: w45 -> [_]
        timing-out: [_] -> w44
        shift-right: [w506] -> _
        shift-left: 1 ("Counter Value") -> [w510]
        shift-left: 0 ("Counter Value") -> [w508]
        shift-right: [w505] -> _
        shift-left: 1 ("Counter Value") -> [w509]
        shift-left: 0 ("Counter Value") -> [w507]
        shift-right: [w489] -> _
        shift-left: 0.0 ("x") -> [w494]
        shift-right: [w491] -> _
        shift-left: 0.0 ("Theta") -> [w502]
        shift-right: [w488] -> _
        shift-left: 0.0 ("y") -> [w493]
        shift-right: [w480] -> _
        shift-left: 0.0 -> [w481]
        stop <- w535 stop-if-true
        w495 = 0.161  # Robot Width
        # "Weird phenomenon, PID returns NaN to duty cycle at the start.\n\nEdit 1: Currently there is one safety mechanism built in, if the output is NaN, Duty Cycle would then be set to 0."
        # "Check if it saturate?\nAnd where the leaks originate from"
        # "Check! The average value should be large when there is no obstacle!"
        # "sBar (cumulative)"
        # "width orignal: 0.1686"
        # "Main Loop"
        n48 = node-c288() -> (w526:i64)  [unwired: 1 in, 1 out]
        n49 = Subtract(x=w510, y=w508) -> (x-y=w503:i32)
        n50 = Subtract(x=w509, y=w507) -> (x-y=w504:i32)
        n51 = To Double Precision Float(number=w526) -> (double precision float=w485:dbl)
        n52 = xnode "Motor 1 Encoder"("error in (no error)"=w498) -> ("Counter Value"=w506:i32, "Counter Direction"=→"Counter Direction":T21, "Overflow?"=→"Overflow?":bool, "error out"=w532:errorcluster)  [unwired: 1 in]
        "Motor 1 Encoder Count" <- w506
        n53 = xnode ("Motor 2 Encoder")("error in (no error)"=w498) -> ("Counter Value"=w505:i32, "Counter Direction"=→"Counter Direction 2":T21, "Overflow?"=→"Overflow? 2":bool, "error out"=w515:errorcluster)  [unwired: 1 in]
        "Motor 2 Encoder Count" <- w505
        n54 = call "DeadReckoning (SubVI).vi"("Theta_0"=w502, "Robot Width"=w495, "y0"=w493, "x0"=w494, "sL"=w503, "sR"=w504) -> ("Theta Actual (rad)"=w490:dbl, "Theta (rad)"=w491:dbl, "y"=w488:dbl, "x"=w489:dbl, "sBar"=w482:dbl)  [unwired: 1 in]
        "x" <- w489
        "Theta Actual (rad)" <- w490
        n55 = shared-variable ".\\LIDAR Data Variables.lvlib\\LIDAR Right y-avg (forward) (m)"() -> (→"LIDAR Right x-avg (m)":dbl)  [unwired: 1 in, 1 out]
        n56 = shared-variable ".\\LIDAR Data Variables.lvlib\\LIDAR Left y-avg (forward) (m)"() -> (→"LIDAR Left x-avg (m)":dbl)  [unwired: 1 in, 1 out]
        n57 = local read "LIDAR LOOP V_RIGHT"() -> (w478:dbl)
        n58 = Add(x=w481, y=w482) -> (x+y=w480:dbl)
        "Total Distance Travelled" <- w480
        n59 = call "CountToDistance (SubVI).vi"("Counter Value"=w506) -> ("Total Distance Travelled (m)"=→"Motor 1 Total Distance":dbl)  [unwired: 10 in]
        n60 = call "Avg Dist To Left Wall (SubVI).vi"() -> ()  [unwired: 12 in]
        n61 = call "CountToDistance (SubVI).vi"("Counter Value"=w505) -> ("Total Distance Travelled (m)"=→"Motor 2 Total Distance":dbl)  [unwired: 10 in]
        n62 = local read "LIDAR LOOP V_LEFT"() -> (w479:dbl)
        n63 = call "SimplePidController (SubVI).vi"("Encoder Count Difference"=w504, "Period of Timed Loop"=w485, "Speed Setpoint"=w478) -> ("Output to Duty Cycle"=w500:dbl, "Output to PWM"=→"Output to PWM 2":dbl, "Speed of Motor"=→"Speed of Motor 2":dbl, "Boolean Output for Motor Driver"=w511:bool)  [unwired: 5 in]
        n64 = call "SimplePidController (SubVI).vi"("Encoder Count Difference"=w503, "Period of Timed Loop"=w485, "Speed Setpoint"=w479) -> ("Output to Duty Cycle"=w501:dbl, "Output to PWM"=→"Output to PWM":dbl, "Speed of Motor"=→"Speed of Motor 1":dbl, "Boolean Output for Motor Driver"=w514:bool)  [unwired: 5 in]
        n65 = shared-variable ".\\Robot Data Variables.lvlib\\Robot Current Heading - Theta Actual (rad)"(w490) -> ()  [unwired: 1 in, 1 out]
        n66 = Not(x=w511) -> (.not. x?=w512:bool)
        n67 = Not(x=w514) -> (.not. x?=w513:bool)
        n68 = xnode "Motor Driver 1 ENB PWM"("error in (no error)"=w498, "Duty Cycle"=w500, "Frequency [Hz]"=10000.0) -> ("error out"=w520:errorcluster)
        n69 = xnode "Motor Driver 1 IN3"("error in (no error)"=w498, "A/DIO2 (Pin 15)"=w512) -> ("error out"=w519:errorcluster)
        n70 = xnode "Motor Driver 1 IN4"("error in (no error)"=w498, "A/DIO3 (Pin 17)"=w511) -> ("error out"=w518:errorcluster)
        n71 = xnode "Motor Driver 1 ENA PWM"("error in (no error)"=w498, "Duty Cycle"=w501, "Frequency [Hz]"=10000.0) -> ("error out"=w527:errorcluster)
        n72 = xnode "Motor Driver 1 IN1"("error in (no error)"=w498, "A/DIO0 (Pin 11)"=w514) -> ("error out"=w530:errorcluster)
        n73 = xnode "Motor Driver 1 IN2"("error in (no error)"=w498, "A/DIO1 (Pin 13)"=w513) -> ("error out"=w529:errorcluster)
        n74 = Negate(x=w488) -> (-x=w486:dbl)
        "y" <- w486
        n75 = Build Array(w489, w486) -> (w487:dbl[])
        n76 = shared-variable ".\\Robot Data Variables.lvlib\\Obs. Avoid. Wall SetPt (m)"() -> (→"Obs. Avoid. Wall SetPt (m)":dbl)  [unwired: 1 in, 1 out]
        n77 = shared-variable ".\\Robot Data Variables.lvlib\\Robot XY Position (m)"(w487) -> ()  [unwired: 1 in, 1 out]
        n78 = Merge Errors(w515, w520, w519, w518) -> (w499:errorcluster)
        n79 = Merge Errors "Merge Errors"(w532, w527, w530, w529, w499) -> (w531:errorcluster)
        n80 = shared-variable ".\\LIDAR Data Variables.lvlib\\Stop VFH Visual"("Stop") -> ()  [unwired: 1 in, 1 out]
        n81 = Or(x=w531, y="Stop") -> (x .or. y?=w535:bool)
        n82 = node-c288() -> ()  [unwired: 1 in, 1 out]
      }
      n83 = while {
        shift-right: [w84] -> _
        shift-left: StateMachineControl."init/pause" ("State") -> [w86]
        stop <- w82 stop-if-true
        n84 = case shown="\"blue uneven surface\"" w86 {
          tunnel: [w91 w135 StateMachineControl."wall tracking w/ obs avoidance" ("State") StateMachineControl."wall tracking w/ obs avoidance" ("State") StateMachineControl."wall tracking w/ obs avoidance" ("State") StateMachineControl."stop robot" ("State") StateMachineControl."go forward fixed dist & stop" ("State") StateMachineControl."wall tracking w/ obs avoidance" ("State") w405 StateMachineControl."init/pause" ("State") StateMachineControl."stop finite state machine" ("State")] -> w84
          frame "init/pause" {
            w87 = 0.0 ("Min Speed")
            n85 = disable-structure shown="Disabled" {
              frame Disabled {
                n86 = local write "Robot Speed"(0.0 ("Robot Speed")) -> ()
              }
              frame Enabled {
              }
            }
            n87 = local write "Wall Tracking Boolean"(TRUE ("Wall Tracking Boolean")) -> ()
            n88 = xnode "Button"() -> ("Value"=w90:bool)  [unwired: 1 in, 1 out]
            n89 = Or(x=w90, y="Go!") -> (x .or. y?=w88:bool)
            n90 = local write "Min Speed"(w87) -> ()
            n91 = local write "Max Speed"(w87) -> ()
            n92 = Select(t=StateMachineControl."go forward fixed dist & continue" ("State"), s=w88, f=StateMachineControl."init/pause" ("State")) -> (s? t:f=w91:T1)
          }
          frame "wall tracking w/ obs avoidance" {
            w175 = FALSE ("LED0")
            # "can set these two to 0 in other states, then when we come back here,\nwe will accelerate again."
            # "note that top speed = min + max"
            # "Code Explanation:\nExample\nFor the yellow tape case, check if the boolean array is exactly TRUE FALSE FALSE using the compound arithmetic in 'AND' mode. If the output result is true, then this should be the only TRUE case. Cascade the result forward with the 'select' operator."
            # "1. Yellow\n2. Red\n3. Green\n4. Blue (to be implemented)"
            # "Comparison functions treat the Boolean value TRUE as greater than the Boolean value FALSE."
            # "incorporate acceleration later"
            n93 = local read "Pixy Output Array"() -> (w141:bool[])
            n94 = shared-variable ".\\Robot Data Variables.lvlib\\Obs. Avoid. Wall SetPt (m)"() -> (w152:dbl)  [unwired: 1 in, 1 out]
            n95 = local read "speed setpoint (m/s)"() -> (w151:dbl)
            n96 = shared-variable ".\\LIDAR Data Variables.lvlib\\LIDAR Left y-avg (side) (m)"() -> (w134:dbl)  [unwired: 1 in, 1 out]
            n97 = local write "Wall Tracking Boolean"(TRUE ("Wall Tracking Boolean")) -> ()
            n98 = Index Array(array=w141, index=0) -> (element=w162:bool)
            n99 = Index Array(array=w141, index=1) -> (element=w161:bool)
            n100 = Index Array(array=w141, index=2) -> (element=w163:bool)
            n101 = Index Array(array=w141, index=3) -> (element=w147:bool)
            n102 = local write "Robot Speed"(w151) -> ()
            n103 = local write "Dist From Wall Setpoint"(w152) -> ()
            n104 = Greater?(x=w134, y=0.56) -> ()  [unwired: 1 out]
            n105 = Equal?(x=w162, y=TRUE) -> (x = y?=w168:bool)
            n106 = Equal?(x=w162, y=FALSE) -> (x = y?=w139:bool)
            n107 = Equal?(x=w161, y=FALSE) -> (x = y?=w138:bool)
            n108 = Equal?(x=w147, y=TRUE) -> (x = y?=w144:bool)
            n109 = Equal?(x=w161, y=TRUE) -> (x = y?=w160:bool)
            n110 = Equal?(x=w163, y=TRUE) -> (x = y?=w159:bool)
            n111 = Equal?(x=w147, y=FALSE) -> (x = y?=w140:bool)
            n112 = Equal?(x=w163, y=FALSE) -> (x = y?=w137:bool)
            n113 = local write "Min Speed"(0.4 ("Min Speed")) -> ()
            n114 = local write "Max Speed"(0.8 ("Max Speed")) -> ()
            n115 = Compound Arithmetic op=AND(w168, w138, w137, w140) -> (w167:bool)
            n116 = Compound Arithmetic op=AND(w139, w160, w137, w140) -> (w158:bool)
            n117 = Select(t=StateMachineControl."yellow zig-zag" ("State"), s=w167, f=StateMachineControl."wall tracking w/ obs avoidance" ("State")) -> (s? t:f=w156:T1)
            n118 = Compound Arithmetic op=AND(w139, w138, w159, w140) -> (w155:bool)
            n119 = Compound Arithmetic op=AND(w144, w139, w138, w137) -> (w143:bool)
            n120 = Select(t=StateMachineControl."red ramp" ("State"), s=w158, f=w156) -> (s? t:f=w153:T1)
            n121 = Select(t=StateMachineControl."green prepare to stop" ("State"), s=w155, f=w153) -> (s? t:f=w136:T1)
            n122 = Select(t=StateMachineControl."blue uneven surface" ("State"), s=w143, f=w136) -> (s? t:f=w135:T1)
            n123 = xnode "LED 4"("LED0"=w175, "LED1"=w175, "LED2"=w175, "LED3"=w175) -> ()  [unwired: 1 in, 1 out]
          }
          frame "yellow zig-zag" {
            # "yellow zig-zag plan (executed via the stacked sequence frames)\n1) when the first yellow tape is detected, go into zig-zag mode.\n2) alternate between minimum and maximum wall-tracking distance per every set time/distance.\n3) go back to normal wall tracking mode after total set time/distance has elapsed."
            n124 = stacked-sequence {
              frame #0 {
                # "mark the current total distance, alternate between different waypoints based on the changes in total distance."
                n125 = local read "Total Distance Travelled"() -> (w220:dbl)
                n126 = local write "Marked Distance"(w220) -> ()
              }
              frame #1 {
                n127 = while {
                  stop <- w222 stop-if-true
                  n128 = local read "Total Distance Travelled"() -> (w224:dbl)
                  n129 = local read "Marked Distance"() -> (w226:dbl)
                  n130 = local write "Dist From Wall Setpoint"(0.1 ("Dist From Wall Setpoint")) -> ()
                  n131 = Add(x=w226, y=0.3) -> (x+y=w223:dbl)
                  n132 = Greater?(x=w224, y=w223) -> (0:w222:bool)
                }
              }
              frame #2 {
                n133 = while {
                  stop <- w228 stop-if-true
                  n134 = local read "Total Distance Travelled"() -> (w230:dbl)
                  n135 = local read "Marked Distance"() -> (w232:dbl)
                  n136 = local write "Dist From Wall Setpoint"(0.45 ("Dist From Wall Setpoint")) -> ()
                  n137 = Add(x=w232, y=0.6) -> (x+y=w229:dbl)
                  n138 = Greater?(x=w230, y=w229) -> (0:w228:bool)
                }
              }
              frame #3 {
                n139 = disable-structure shown="Disabled" {
                  frame Disabled {
                    n140 = while {
                      stop <- w234 stop-if-true
                      n141 = local read "Total Distance Travelled"() -> (w236:dbl)
                      n142 = local read "Marked Distance"() -> (w238:dbl)
                      n143 = local write "Dist From Wall Setpoint"(0.1 ("Dist From Wall Setpoint")) -> ()
                      n144 = Add(x=w238, y=1.2) -> (x+y=w235:dbl)
                      n145 = Greater?(x=w236, y=w235) -> (0:w234:bool)
                    }
                  }
                  frame Enabled {
                  }
                }
              }
            }
            n146 = local write "Robot Speed"(0.35 ("Robot Speed")) -> ()
            n147 = local write "Min Speed"(0.15 ("Min Speed")) -> ()
            n148 = local write "Max Speed"(0.0 ("Max Speed")) -> ()
            n149 = xnode "LED"("LED0"=TRUE) -> ()  [unwired: 1 in, 1 out]
          }
          frame "blue uneven surface" {
            # "To be implemented:\n\nOnce blue uneven surface is detected, slow down immediately.\n\nThen continue at the slower speed while wall-tracking, then restore restore back to normal speed after finishing the uneven surface section."
            n150 = stacked-sequence {
              frame #0 {
                n151 = local read "Total Distance Travelled"() -> (w277:dbl)
                n152 = local write "Marked Distance"(w277) -> ()
              }
              frame #1 {
                n153 = while {
                  stop <- w278 stop-if-true
                  n154 = local read "Total Distance Travelled"() -> (w280:dbl)
                  n155 = local read "Marked Distance"() -> (w282:dbl)
                  n156 = Add(x=w282, y=0.9) -> (x+y=w279:dbl)
                  n157 = Greater?(x=w280, y=w279) -> (0:w278:bool)
                }
              }
            }
            n158 = local write "Dist From Wall Setpoint"(0.27 ("Dist From Wall Setpoint")) -> ()
            n159 = local write "Robot Speed"(0.3 ("Robot Speed")) -> ()
          }
          frame "red ramp" {
            n160 = stacked-sequence {
              frame #0 {
                # "Use the following quantities:\n1) Total distance travelled\n2) Theta actual (current heading)\n3) LIDAR measured angle\n\nSet the Marked Heading such that the robot will go straight over the ramp."
                n161 = local read "Total Distance Travelled"() -> (w292:dbl)
                n162 = local read "LIDAR Measured Angle"() -> (w290:dbl)
                n163 = local read "Theta Actual (rad)"() -> (w293:dbl)
                n164 = expression code="(x/pi)*180.0" "radians to degrees"(w293) -> (w291:dbl)
                n165 = Subtract(x=w291, y=w290) -> (x-y=w289:dbl)
                n166 = local write "Marked Distance"(w292) -> ()
                n167 = local write "Marked Heading"(w289) -> ()
              }
              frame #1 {
                n168 = while {
                  stop <- w294 stop-if-true
                  # "Tell the robot to go straight for 'x' metres."
                  # "Now, have the robot go over the ramp. Then return to the normal wall tracking state."
                  n169 = local read "Marked Heading"() -> (w299:dbl)
                  n170 = local read "Total Distance Travelled"() -> (w296:dbl)
                  n171 = local read "Marked Distance"() -> (w298:dbl)
                  n172 = local write "Robot Heading"(w299) -> ()
                  n173 = Add(x=w298, y=0.8) -> (x+y=w295:dbl)
                  n174 = Greater?(x=w296, y=w295) -> (0:w294:bool)
                }
              }
            }
            n175 = local write "Wall Tracking Boolean"(FALSE ("Wall Tracking Boolean")) -> ()
            n176 = local write "Robot Speed"(0.4 ("Robot Speed")) -> ()
            n177 = local write "Min Speed"(0.3 ("Min Speed")) -> ()
            n178 = local write "Max Speed"(0.0 ("Max Speed")) -> ()
            n179 = xnode "LED 2"("LED1"=TRUE) -> ()  [unwired: 1 in, 1 out]
          }
          frame "green prepare to stop" {
            # "It is an extrememly bad idea to reset the encoder counter!\nTry noting down the total distance travelled instead."
            n180 = stacked-sequence {
              frame #0 {
                n181 = local read "Total Distance Travelled"() -> (w337:dbl)
                n182 = local read "Theta Actual (rad)"() -> (w339:dbl)
                n183 = expression code="(x/pi)*180.0" "radians to degrees"(w339) -> (w338:dbl)
                n184 = local write "Marked Distance"(w337) -> ()
                n185 = local write "Marked Heading"(w338) -> ()
              }
              frame #1 {
                n186 = while {
                  stop <- w340 stop-if-true
                  n187 = local read "Marked Heading"() -> (w346:dbl)
                  n188 = local read "Total Distance Travelled"() -> (w341:dbl)
                  n189 = local read "Marked Distance"() -> (w344:dbl)
                  n190 = local write "Wall Tracking Boolean"(FALSE ("Wall Tracking Boolean")) -> ()
                  n191 = local write "Robot Heading"(w346) -> ()
                  n192 = local write "Robot Speed"(0.3 ("Robot Speed")) -> ()
                  n193 = Add(x=w344, y=0.37) -> (x+y=w342:dbl)
                  n194 = Greater?(x=w341, y=w342) -> (0:w340:bool)
                }
              }
              frame #2 {
                n195 = local write "Robot Speed"(0.0 ("Robot Speed")) -> ()
              }
            }
            n196 = xnode "LED 3"("LED2"=TRUE) -> ()  [unwired: 1 in, 1 out]
          }
          frame "note down current distance" {
            # "DO NOT DELETE THIS STATE! It holds the Marked Heading and Marked Distance variables which are used elsewhere."
            # "This method does not fully work because when the encoder counts are different, we still need to reset the direction/angle of the robot."
            n197 = local read "Total Distance Travelled"() -> (w384:dbl)
            n198 = local read "Theta Actual (rad)"() -> (w386:dbl)
            n199 = expression code="(x/pi)*180.0" "radians to degrees"(w386) -> (w385:dbl)
            n200 = local write "Marked Distance"(w384) -> ()
            n201 = local write "Marked Heading"(w385) -> ()
          }
          frame "go forward fixed dist & continue" {
            w388 = 0.0 ("Min Speed")
            n202 = stacked-sequence {
              frame #0 {
                n203 = local read "Total Distance Travelled"() -> (w392:dbl)
                n204 = local read "Theta Actual (rad)"() -> (w391:dbl)
                n205 = expression code="(x/pi)*180.0" "radians to degrees"(w391) -> (w390:dbl)
                n206 = local write "Marked Distance"(w392) -> ()
                n207 = local write "Marked Heading"(w390) -> ()
              }
              frame #1 {
                n208 = while {
                  stop <- w393 stop-if-true
                  n209 = local read "Total Distance Travelled"() -> (w394:dbl)
                  n210 = local read "Marked Heading"() -> (w398:dbl)
                  n211 = local read "Marked Distance"() -> (w396:dbl)
                  n212 = Add(x=w396, y=0.2) -> (x+y=w395:dbl)
                  n213 = local write "Marked Heading"(w398) -> ()
                  n214 = local write "Robot Speed"(0.3 ("Robot Speed")) -> ()
                  n215 = Greater?(x=w394, y=w395) -> (0:w393:bool)
                }
              }
            }
            n216 = local write "Max Speed"(w388) -> ()
            n217 = local write "Min Speed"(w388) -> ()
          }
          frame "go forward fixed dist & stop" {
            # "stop robot once it has moved 'x' m past the first green tape"
            n218 = local read "Marked Heading"() -> (w401:dbl)
            n219 = local write "Wall Tracking Boolean"(FALSE ("Wall Tracking Boolean")) -> ()
            n220 = local read "Total Distance Travelled"() -> (w400:dbl)
            n221 = local read "Marked Distance"() -> (w403:dbl)
            n222 = local write "Robot Heading"(w401) -> ()
            n223 = local write "Robot Speed"(0.1 ("Robot Speed")) -> ()
            n224 = Add(x=w403, y=0.4) -> (x+y=w402:dbl)
            n225 = Greater?(x=w400, y=w402) -> (0:w408:bool)
            n226 = Select(t=StateMachineControl."stop robot" ("State"), s=w408, f=StateMachineControl."go forward fixed dist & stop" ("State")) -> (s? t:f=w405:T1)
          }
          frame "stop robot" {
            n227 = local write "Robot Speed"(0.0 ("Robot Speed")) -> ()
          }
          frame "stop finite state machine" {
          }
        }
        n228 = local read "Stop"() -> (w81:bool)
        n229 = Equal?(x=w86, y=StateMachineControl."stop finite state machine") -> (x = y?=w83:bool)
        n230 = Or(x=w81, y=w83) -> (x .or. y?=w82:bool)
      }
      n231 = node-c288() -> (w24:T2)  [unwired: 4 in]
      n232 = while {
        shift-right: [w75] -> w22
        shift-left: w25 -> [w77]
        tunnel: w26 -> [w78]
        stop <- w79 stop-if-true
        n233 = call "PixySigDetect.vi"("error in (no error)"=w77, "Signature Number"=u8 255, "VISA resource name"=w78) -> ("error out"=w76:errorcluster, "Data"=w73:string)  [unwired: 5 in, 2 out]
        n234 = call "PixyAllDetect.vi"("error in (no error)"=w76, "String"=w73) -> ("error out"=w75:errorcluster, "output array"=→"Pixy Output Array":bool[])  [unwired: 8 in]
        n235 = local read "Stop"() -> (w79:bool)
        n236 = Wait (ms)(milliseconds to wait=u32 50) -> ()  [unwired: 1 out]
      }
      n237 = timed-loop {
        timing: w24 -> [_]
        timing-out: [_] -> w23
        shift-right: [w61] -> _
        shift-left: 1.0 ("Theta Actual (rad)") -> [w65]
        shift-right: [w48] -> _
        shift-left: 0.0 ("Theta Actual (rad)") -> [w64]
        stop <- w67 stop-if-true
        w52 = 1.0 ("y")
        # "Min Speed and Max Speed to be set by the finite state machine."
        # "speed setpoint (m/s)"
        # "Actual Top Speed = Min Speed + Max Speed"
        # "Theta Actual (rad)"
        # "Acceleration"
        # "Acceleration"
        n238 = node-c288() -> ()  [unwired: 1 in, 1 out]
        n239 = local read "Theta Actual (rad)"() -> (w48:dbl)
        n240 = Increment(x=w65) -> (x+1=w62:dbl)
        n241 = local read "Max Speed"() -> (w47:dbl)
        n242 = Divide(x=w47, y=0.015) -> (x/y=w57:dbl)
        n243 = Subtract(x=w48, y=w64) -> (x-y=w63:dbl)
        n244 = Absolute Value(x=w63) -> (abs(x)=w60:dbl)
        n245 = Max & Min(x=w62, y=w57) -> (min(x,y)=w55:dbl)  [unwired: 1 out]
        n246 = expression code="(x/pi)*180.0" "radians to degrees"(w60) -> (w59:dbl)
        n247 = Divide(x=w59, y=60.0) -> (x/y=w51:dbl)
        n248 = Max & Min(x=w52, y=w51) -> (min(x,y)=w50:dbl)  [unwired: 1 out]
        n249 = Subtract(x=w52, y=w50) -> (x-y=w53:dbl)
        n250 = Multiply(x=w53, y=w55) -> (x*y=w61:dbl)
        n251 = local read "Min Speed"() -> (w46:dbl)
        n252 = Multiply(x=w61, y=0.015) -> (x*y=w58:dbl)
        n253 = Add(x=w58, y=w46) -> (x+y=→"speed setpoint (m/s)":dbl)
        n254 = local read "Stop"() -> (w67:bool)
        n255 = node-c288() -> ()  [unwired: 1 in, 1 out]
      }
      n256 = call "VFH Visualization.vi"() -> ()  [unwired: 3 in]
      n257 = node-c288(w23) -> ()  [unwired: 1 out]
      n258 = node-c288(w44) -> (w41:errorcluster)
      n259 = Merge Errors(w41, w40, w30, w22) -> (w42:errorcluster)
    }
    frame #2 {
      # "Close"
      n260 = VISA Close(VISA resource name=w847) -> ()  [unwired: 1 in, 1 out]
      n261 = call <vilib>:"Reset myRIO.vi"("error in (no error)"=w846) -> ("error out"=→"Error Out":errorcluster)  [unwired: 10 in]
    }
  }
